vi "ACT_Loop.vi"() -> ()   [LabVIEW 2023, in "Thor-SwerveDrive_ACT.lvlib"]
uses:
  Thor-SwerveDrive_ACT.lvlib
  roboRIO Utilities/Global_STOP.vi
  ENUM_ACT_Action.ctl
  ENUM_ACT_State.ctl
  Global_CMD_ACT_Data In.vi
  Global_ACT_Data Out.vi
  Cluster_CMD_ACT_Data.ctl
  <vilib>/Rock Robotics/WPI/MotorControl/WPI_MotorControlType.ctl
  <vilib>/Rock Robotics/SystemInterfaces/DIO/FPGA_DIOPWMChannel.ctl
  <vilib>/Rock Robotics/WPI/PWM/WPI_PWMDeadband.ctl
  <vilib>/Rock Robotics/SystemInterfaces/DIO/FPGA_DIOChannel.ctl
  <vilib>/Rock Robotics/WPI/MotorControl/WPI_MotorControlDeviceRef.ctl
  Shared Code/TypeDefs/ENUM_Motor Index.ctl
  Shared Code/TypeDefs/ENUM_Swerve_CMD_Mode Select.ctl
  Type Defs/ENUM_Steer Mode Select.ctl
  Shared Code/TypeDefs/Cluster_CMD_Direction Data.ctl
  Shared Code/TypeDefs/Level_Velocity plus-minus 1.ctl
  Shared Code/TypeDefs/Dial_Compase heading unit circle CCW positive.ctl
  Shared Code/TypeDefs/Cluster_Module Velocity-Direction-Rotations.ctl
  Shared Code/TypeDefs/Cluster_Swerve 4 Steer and Velocity.ctl
  Shared Code/TypeDefs/Cluster_X-Y.ctl
  Type Defs/Cluster_Length and Width.ctl
  PigeonIMU/Global_SEN_Data Out.vi
  PigeonIMU/PigeonIMU_SEN.lvlib
  <vilib>/Rock Robotics/WPI/ThirdParty/Phoenix-LabVIEW/CANCoder/Controls/CTRE_Phoenix_CANcoder_DeviceRef.ctl
  <vilib>/Rock Robotics/WPI/ThirdParty/Phoenix-LabVIEW/Motor Controller/Controls/CTRE_Phoenix_MotorControl_ControlMode.ctl
  <vilib>/Rock Robotics/WPI/ThirdParty/Phoenix-LabVIEW/Motor Controller/Get/CTRE_Phoenix_MotorController_GetSelectedSensorData.vi
  Shared Code/TypeDefs/Cluster_Module Specific Config Data.ctl
  <vilib>/Rock Robotics/WPI/ThirdParty/Phoenix-LabVIEW/Motor Controller/Controls/CTRE_Phoenix_MotorControl_TalonFXInvertType.ctl
  <vilib>/Rock Robotics/WPI/ThirdParty/Phoenix-LabVIEW/Motor Controller/Controls/CTRE_Phoenix_MotorControl_NeutralMode.ctl
  Shared Code/TypeDefs/Cluster_Enable-Value DBL.ctl
  Shared Code/TypeDefs/Cluster_Swerve Module Drive Config Data.ctl
  Shared Code/TypeDefs/Cluster_PID Gains.ctl
  Shared Code/TypeDefs/Cluster_High-Low.ctl
  Shared Code/TypeDefs/Cluster_PID Config.ctl
  Shared Code/TypeDefs/Cluster_Swerve Module Azimuth Config Data.ctl
  Shared Code/TypeDefs/Cluster_Motion Magic Parameters.ctl
  Type Defs/NUM_Rotate Input.ctl
  Shared Code/TypeDefs/Cluster_Swerve Specific Data.ctl
  4adeeee4-476d-45d4-a5a4-571a9ae37a33.vi
  2c7c5537-7bdd-4d59-ad4f-3c8ee235c6a6.vi
  807b9100-2ea1-4d3f-8102-f0ab848f34e3.vi
  19b81104-80f8-498e-bad8-80b5a07e1603.vi
  e1bb1583-82cd-4173-857f-54dda67d13bd.vi
  9120009a-4733-4867-ae1d-0cf0254934b1.vi
  e3bd2e4a-1335-45b3-b961-e3cd167d7084.vi
  9ce11db1-6321-4cd7-bc1a-63dd18007c8f.vi
  Shared Code/TypeDefs/Cluster_FWD  REV Values.ctl
  Shared Code/TypeDefs/Cluster_Config Motor Output.ctl
  8c0680db-f6e2-43d9-8911-a02d1c4f353c.vi
  f7ff1910-59a6-4a5b-a4bc-add152f69b28.vi
  140e803e-7328-4941-96e6-52945a01db81.vi
  4178fa8d-7c82-4047-aba6-40e6de057a6a.vi
  2d114f5c-e136-49d5-a090-2a73a4719927.vi
  136452eb-6d18-483f-b532-0de35bf94788.vi
  Shared Code/TypeDefs/Cluster_Config_AutoRotate Data.ctl
  Shared Code/TypeDefs/Cluster_Config_AutoDrive Data.ctl
  Shared Code/TypeDefs/Cluster_Config_Balance Data.ctl
  eab307ff-2afe-4630-93b3-566b0cf5e78a.vi
  51c25ad4-39a0-4a24-89e8-b12740a342fe.vi
  Type Defs/Cluster_Pigeon Tilt Data.ctl
  Shared Code/TypeDefs/ENUM_Tilt State.ctl
  Shared Code/TypeDefs/Cluster_Config_SwerveParam Steer.ctl
  Shared Code/TypeDefs/Cluster_Config_SwerveParam Drive.ctl
  Shared Code/TypeDefs/Cluster_Config_Swerve Drive Parameters.ctl
  <vilib>/Rock Robotics/WPI/ThirdParty/Phoenix-LabVIEW/Motor Controller/Get/CTRE_Phoenix_MotorController_GetVoltage.vi
  <vilib>/Rock Robotics/WPI/ThirdParty/Phoenix-LabVIEW/CANCoder/Get/CTRE_Phoenix_CANcoder_GetSensorData.vi
  Shared Code/TypeDefs/Dial_Actual Direction.ctl
  Shared Code/TypeDefs/Cluster_Module Actual Settings.ctl
  Shared Code/TypeDefs/Cluster_Swerve Actual Settings.ctl
panel:
  out "x-y":dbl
  out "Velocity":dbl[](array[numeric])
  out "Velocity Out":dbl
  out "At Target":bool
  out "State":T1
  out "Balanced":bool
  in  "Balance Config":T2={"BalancePID Ver"=0, "PID"={"Gains"={"P"=4.0, "I"=0.0, "D"=50.0, "F"=0.0}, "Error Allowed"={"High"=0.01, "Low"=-0.01}, "I Zone"={"High"=10.0, "Low"=-10.0}, "Max Out"={"FWD"=0.44, "REV"=-0.44}, "Max I Accu"={"High"=100000.0, "Low"=-100000.0}, "CL Ramp Rate (S)"=0.01}} {"PID"."Max I Accu"."Low" format="%#.8f"; "PID"."Max I Accu"."High" format="%#.8f"; "PID"."Gains"."F" format="%#.8f"; "PID"."Gains"."D" format="%#.8f"; "PID"."Gains"."I" format="%#.8f"; "PID"."Gains"."P" format="%#.8f"; "PID"."Error Allowed"."Low" format="%#.8f"; "PID"."Error Allowed"."High" format="%#.8f"; "PID"."I Zone"."Low" format="%#.8f"; "PID"."I Zone"."High" format="%#.8f"; "PID"."Max Out"."REV" format="%.2f"; "PID"."Max Out"."FWD" format="%.2f"}
  out "At Angle":bool
  out "At Position":bool
  in  "Auto Rotate Config":T7={"AutoRotatePID Ver"=0, "PID Config"={"Gains"={"P"=0.005, "I"=0.001, "D"=0.0, "F"=0.0}, "Error Allowed"={"High"=0.05, "Low"=-0.05}, "I Zone"={"High"=0.25, "Low"=-0.25}, "Max Out"={"FWD"=1.0, "REV"=-1.0}, "Max I Accu"={"High"=100000.0, "Low"=-100000.0}, "CL Ramp Rate (S)"=0.002}} {"PID Config"."Max I Accu"."Low" format="%#.8f"; "PID Config"."Max I Accu"."High" format="%#.8f"; "PID Config"."Gains"."F" format="%#.8f"; "PID Config"."Gains"."D" format="%#.8f"; "PID Config"."Gains"."I" format="%#.8f"; "PID Config"."Gains"."P" format="%#.8f"; "PID Config"."Error Allowed"."Low" format="%#.8f"; "PID Config"."Error Allowed"."High" format="%#.8f"; "PID Config"."I Zone"."Low" format="%#.8f"; "PID Config"."I Zone"."High" format="%#.8f"; "PID Config"."Max Out"."REV" format="%.2f"; "PID Config"."Max Out"."FWD" format="%.2f"}
  out "PID Enabled":bool
  out "Auto Drive error":dbl
  in  "Auto PID Config":T8={"AutoDrivePID Ver"=0, "PID Config"={"Gains"={"P"=0.08, "I"=0.0, "D"=0.0, "F"=0.0}, "Error Allowed"={"High"=1.0, "Low"=-1.0}, "I Zone"={"High"=1.0, "Low"=-1.0}, "Max Out"={"FWD"=0.4, "REV"=-0.4}, "Max I Accu"={"High"=100000.0, "Low"=-100000.0}, "CL Ramp Rate (S)"=0.002}} {"PID Config"."Max I Accu"."Low" format="%#.8f"; "PID Config"."Max I Accu"."High" format="%#.8f"; "PID Config"."Gains"."F" format="%#.8f"; "PID Config"."Gains"."D" format="%#.8f"; "PID Config"."Gains"."I" format="%#.8f"; "PID Config"."Gains"."P" format="%#.8f"; "PID Config"."Error Allowed"."Low" format="%#.8f"; "PID Config"."Error Allowed"."High" format="%#.8f"; "PID Config"."I Zone"."Low" format="%#.8f"; "PID Config"."I Zone"."High" format="%#.8f"; "PID Config"."Max Out"."REV" format="%.2f"; "PID Config"."Max Out"."FWD" format="%.2f"}
  in  "Reset Distance":bool
  out "Calculated Position ft":dbl
  in  "Read Saved Config":bool
  out "Current Time":timestamp
  in  "Update Config":bool
  in  "Module Specific Data":T9={"SpecificData Ver"=0, "Data"=[{"Motor Pos"=enum."Left-Front", "CAN Bus"="", "Drive ID"=5, "Azimuth ID"=1, "CanCoder ID"=1, "CanCoder Offset"=14.502}, {"Motor Pos"=enum."Right-Front", "CAN Bus"="", "Drive ID"=6, "Azimuth ID"=2, "CanCoder ID"=2, "CanCoder Offset"=166.816}, {"Motor Pos"=enum."Right-Back", "CAN Bus"="", "Drive ID"=7, "Azimuth ID"=3, "CanCoder ID"=3, "CanCoder Offset"=50.273}, {"Motor Pos"=enum."Left-Back", "CAN Bus"="", "Drive ID"=8, "Azimuth ID"=4, "CanCoder ID"=4, "CanCoder Offset"=332.842}]}
  in  "Azimuth Config Data":T12={"ModuleAzimuth Ver"=0, "Output"={"Type"=enum."Counter-Clockwise", "Neutral"=enum."EEPROMSetting", "Max"={"FWD"=0.0, "REV"=1.0}, "Min"={"FWD"=0.0, "REV"=0.0}, "OL Ramp Rate (S)"=0.0, "Dead Band"=0.0}, "CL"={"Gains"={"P"=1.0, "I"=0.01, "D"=0.0, "F"=0.0}, "Error Allowed"={"High"=0.0, "Low"=0.0}, "I Zone"={"High"=10000.0, "Low"=-1000.0}, "Max Out"={"FWD"=1.0, "REV"=-1.0}, "Max I Accu"={"High"=10.0, "Low"=-10.0}, "CL Ramp Rate (S)"=0.0}, "MM"={"Cruise Velocity"=5000, "Acceleration"=5000}} {"Output"."Min"."REV" format="%.2f"; "Output"."Min"."FWD" format="%.2f"; "Output"."Max"."REV" format="%.2f"; "Output"."Max"."FWD" format="%.2f"; "CL"."Max I Accu"."Low" format="%#.8f"; "CL"."Max I Accu"."High" format="%#.8f"; "CL"."Gains"."F" format="%#.8f"; "CL"."Gains"."D" format="%#.8f"; "CL"."Gains"."I" format="%#.8f"; "CL"."Gains"."P" format="%#.8f"; "CL"."Error Allowed"."Low" format="%#.8f"; "CL"."Error Allowed"."High" format="%#.8f"; "CL"."I Zone"."Low" format="%#.8f"; "CL"."I Zone"."High" format="%#.8f"; "CL"."Max Out"."REV" format="%.2f"; "CL"."Max Out"."FWD" format="%.2f"}
  in  "Drive Config Data":T17={"ModuleDrive Ver"=0, "Output"={"Type"=enum."Counter-Clockwise", "Neutral"=enum."EEPROMSetting", "Max"={"FWD"=0.0, "REV"=0.0}, "Min"={"FWD"=0.0, "REV"=0.0}, "OL Ramp Rate (S)"=0.0, "Dead Band"=0.0}, "CL"={"Gains"={"P"=1.0, "I"=0.01, "D"=0.0, "F"=0.0}, "Error Allowed"={"High"=0.1, "Low"=-0.1}, "I Zone"={"High"=10.0, "Low"=-10.0}, "Max Out"={"FWD"=100.0, "REV"=-100.0}, "Max I Accu"={"High"=0.0, "Low"=0.0}, "CL Ramp Rate (S)"=0.0}, "VoltageComp"={"Enable"=FALSE, "Value"=0.0}} {"Output"."Min"."REV" format="%.2f"; "Output"."Min"."FWD" format="%.2f"; "Output"."Max"."REV" format="%.2f"; "Output"."Max"."FWD" format="%.2f"; "VoltageComp"."Value" format="%.1g"; "CL"."Max I Accu"."Low" format="%#.8f"; "CL"."Max I Accu"."High" format="%#.8f"; "CL"."Gains"."F" format="%#.8f"; "CL"."Gains"."D" format="%#.8f"; "CL"."Gains"."I" format="%#.8f"; "CL"."Gains"."P" format="%#.8f"; "CL"."Error Allowed"."Low" format="%#.8f"; "CL"."Error Allowed"."High" format="%#.8f"; "CL"."I Zone"."Low" format="%#.8f"; "CL"."I Zone"."High" format="%#.8f"; "CL"."Max Out"."REV" format="%.2f"; "CL"."Max Out"."FWD" format="%.2f"}
  out "Drive Control Mode":T19 items=["PercentOutput"=0, "Position"=1, "Velocity"=2, "Current"=3, "Follower"=5, "MotionProfile"=6, "MotionMagic"=7, "MotionProfileArc"=10, "Disabled"=15]
  out "MOTOR-POSITION":dbl[](array[numeric])
  out "CAN-POSITION":dbl[](array[numeric])
  out "RAW":dbl[](array[numeric])
  out "Yaw":T20 scale format="%.3f"
  out "Swerve SET Actual":T21 {"Back Right"."Direction" scale format="%.3f"; "Back Right"."Velocity" format="%.2f"; "Back Left"."Direction" scale format="%.3f"; "Back Left"."Velocity" format="%.2f"; "Front Left"."Direction" scale format="%.3f"; "Front Left"."Velocity" format="%.2f"; "Front Right"."Direction" scale format="%.3f"; "Front Right"."Velocity" format="%.2f"}
  out "calc time":dbl
  out "Swerve Set":T24 {"Back Right"."Angle" scale format="%.3f"; "Back Right"."Velocity" scale=-1.0..1.0 scale format="%.1f"; "Back Left"."Angle" scale format="%.3f"; "Back Left"."Velocity" scale=-1.0..1.0 scale format="%.1f"; "Front Left"."Angle" scale format="%.3f"; "Front Left"."Velocity" scale=-1.0..1.0 scale format="%.1f"; "Front Right"."Angle" scale format="%.3f"; "Front Right"."Velocity" scale=-1.0..1.0 scale format="%.1f"}
  out "Max Velocity(CP100ms)":dbl=200.0
  out "Steer Mode":T27
  out "Max Tranlation FPS":dbl=2.0
  out "Calculated Position Values":i32[](array[numeric])
  in  "Stream":bool
  out "Input CMD":T28 {"Auto Angle" scale format="%.3f"; "Direction"."Rotate(Yaw) CCW 1 CW -1" scale=1.0..-1.0; "Direction"."Traverse"."Angle" scale format="%.3f"; "Direction"."Traverse"."Velocity" scale=-1.0..1.0 scale format="%.1f"}
  out "Cycle Time (S)":dbl format="%.3g"
  # "Tune Output\nto 1023 Max"
  # "Tune to Output\nto 1023 Max"
  # "\"Front\" of Robot"
  # "X"
  # "+CCW"
  # "Y"
  # "(0,0)"
  # "\"Front\" of Robot"
  # "Right Hand Rule"
  # "X"
  # "+CCW"
  # "Y"
  # "(0,0)"
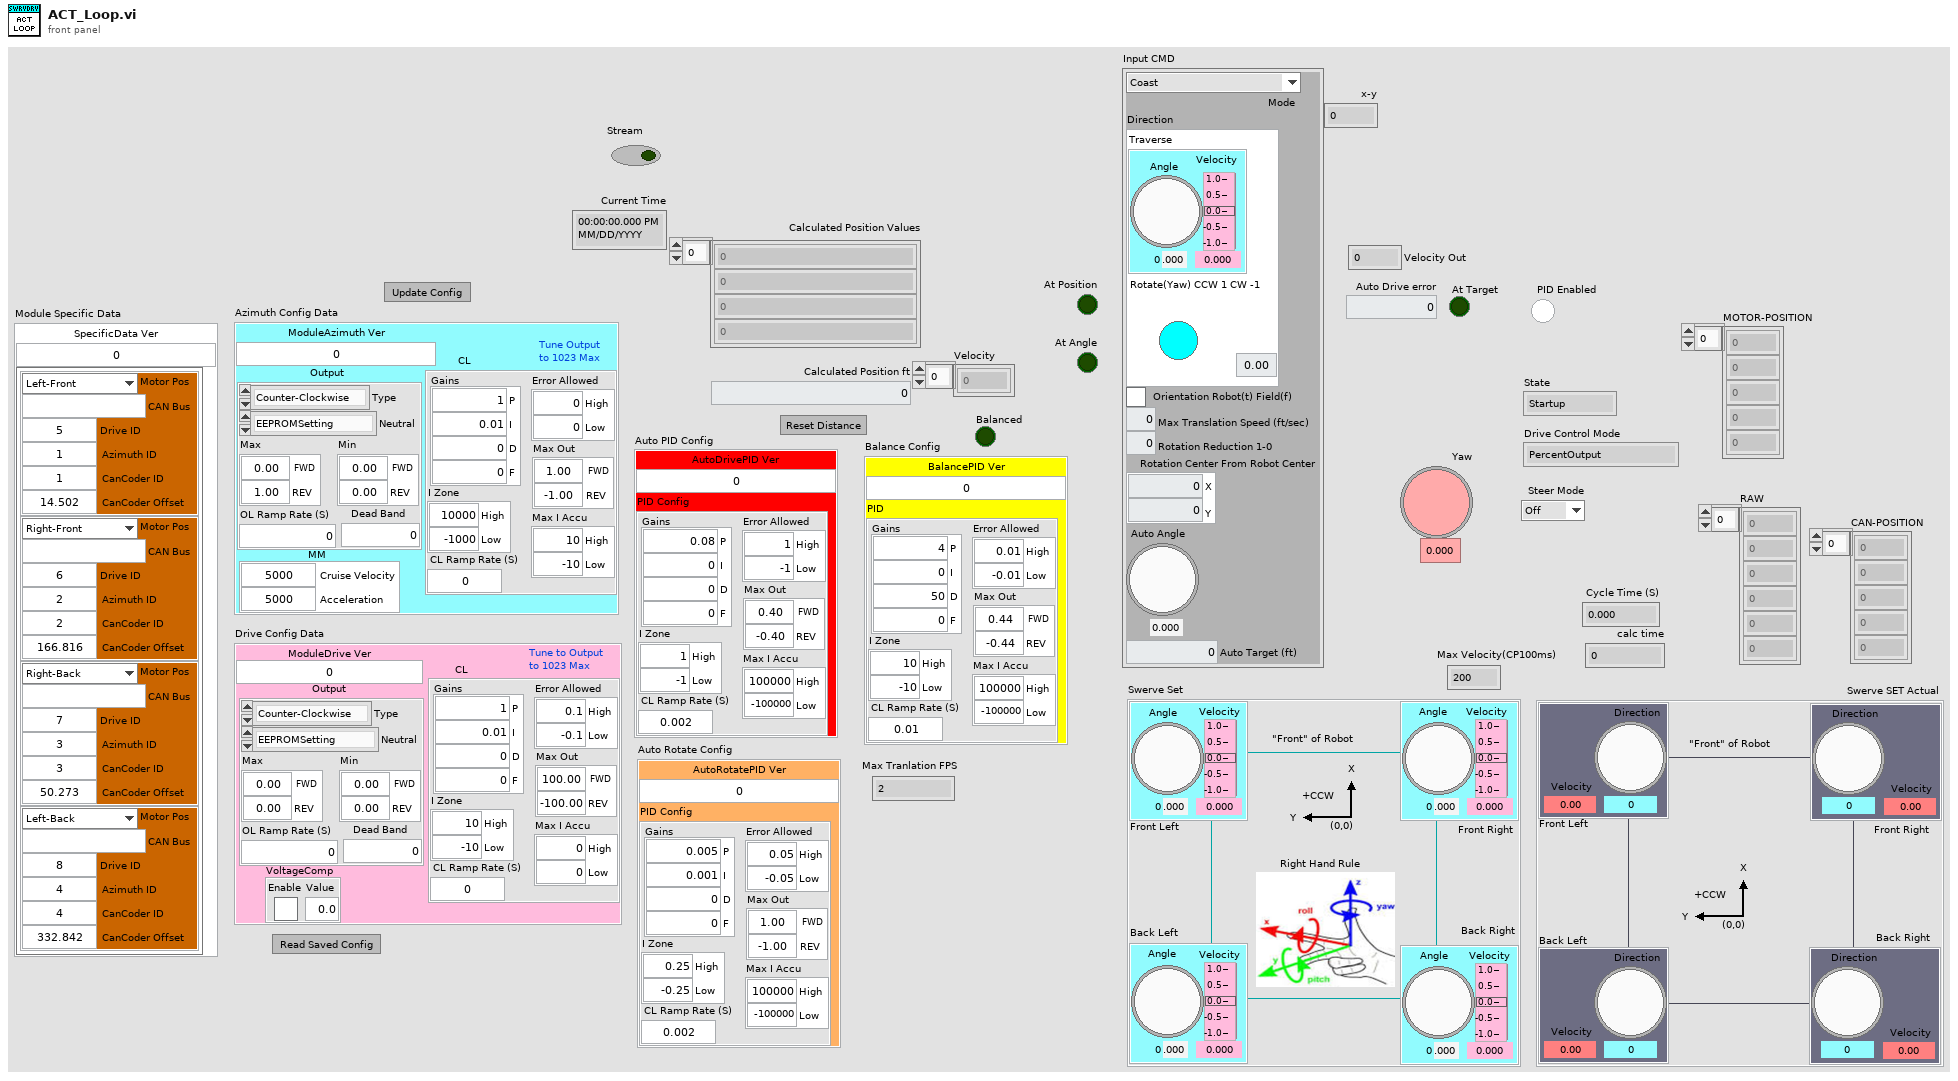
[diagram p1: front panel]
types:
  T1 = typedef "Thor-SwerveDrive_ACT.lvlib/ENUM_ACT_State.ctl" = enum16{"Startup", "Configuring", "Moving", "Coasting", "Shutdown", "Autoing", "Balancing", "Braking", "Locking Wheels"}
  T2 = typedef "Cluster_Config_Balance Data.ctl" = cluster{"BalancePID Ver":u64, "PID":T3}
  T3 = typedef "Cluster_PID Config.ctl" = cluster{"Gains":T4, "Error Allowed":T5, "I Zone":T5, "Max Out":T6, "Max I Accu":T5, "CL Ramp Rate (S)":dbl}
  T4 = typedef "Cluster_PID Gains.ctl" = cluster{"P":dbl, "I":dbl, "D":dbl, "F":dbl}
  T5 = typedef "Cluster_High-Low.ctl" = cluster{"High":dbl, "Low":dbl}
  T6 = typedef "Cluster_FWD  REV Values.ctl" = cluster{"FWD":dbl, "REV":dbl}
  T7 = typedef "Cluster_Config_AutoRotate Data.ctl" = cluster{"AutoRotatePID Ver":u64, "PID Config":T3}
  T8 = typedef "Cluster_Config_AutoDrive Data.ctl" = cluster{"AutoDrivePID Ver":u64, "PID Config":T3}
  T9 = typedef "Cluster_Swerve Specific Data.ctl" = cluster{"SpecificData Ver":u64, "Data":T10[]}
  T10 = typedef "Cluster_Module Specific Config Data.ctl" = cluster{"Motor Pos":T11, "CAN Bus":string, "Drive ID":u8, "Azimuth ID":u8, "CanCoder ID":u8, "CanCoder Offset":dbl}
  T11 = typedef "ENUM_Motor Index.ctl" = enum16{"Left-Front", "Right-Front", "Left-Back", "Right-Back"}
  T12 = typedef "Cluster_Swerve Module Azimuth Config Data.ctl" = cluster{"ModuleAzimuth Ver":u64, "Output":T13, "CL":T3, "MM":T16}
  T13 = typedef "Cluster_Config Motor Output.ctl" = cluster{"Type":T14, "Neutral":T15, "Max":T6, "Min":T6, "OL Ramp Rate (S)":dbl, "Dead Band":dbl}
  T14 = typedef "CTRE_Phoenix_MotorControl_TalonFXInvertType.ctl" = enum16{"Counter-Clockwise", "Clockwise"}
  T15 = typedef "CTRE_Phoenix_MotorControl_NeutralMode.ctl" = enum8{"EEPROMSetting", "Override to Coast", "Override to Brake"}
  T16 = typedef "Cluster_Motion Magic Parameters.ctl" = cluster{"Cruise Velocity":i32, "Acceleration":i32}
  T17 = typedef "Cluster_Swerve Module Drive Config Data.ctl" = cluster{"ModuleDrive Ver":u64, "Output":T13, "CL":T3, "VoltageComp":T18}
  T18 = typedef "Cluster_Enable-Value DBL.ctl" = cluster{"Enable":bool, "Value":dbl}
  T19 = typedef "CTRE_Phoenix_MotorControl_ControlMode.ctl" = u16
  T20 = typedef "Dial_Compase heading unit circle CCW positive.ctl" = dbl
  T21 = typedef "Cluster_Swerve Actual Settings.ctl" = cluster{"Front Right":T22, "Front Left":T22, "Back Left":T22, "Back Right":T22}
  T22 = typedef "Cluster_Module Actual Settings.ctl" = cluster{"Velocity":dbl, "Direction":T23, "Encoder":dbl}
  T23 = typedef "Dial_Actual Direction.ctl" = dbl
  T24 = typedef "Cluster_Swerve 4 Steer and Velocity.ctl" = cluster{"Front Right":T25, "Front Left":T25, "Back Left":T25, "Back Right":T25}
  T25 = typedef "Cluster_Module Velocity-Direction-Rotations.ctl" = cluster{"Velocity":T26, "Angle":T20, "Rotations Count":dbl}
  T26 = typedef "Level_Velocity plus-minus 1.ctl" = dbl
  T27 = typedef "ENUM_Steer Mode Select.ctl" = enum16{"Off", "Hold", "Steer"}
  T28 = typedef "Thor-SwerveDrive_ACT.lvlib/Cluster_CMD_ACT_Data.ctl" = cluster{"Mode":T29, "Direction":T30, "Orientation Robot(t) Field(f)":bool, "Max Translation Speed (ft/sec)":dbl, "Rotation Reduction 1-0":dbl, "Rotation Center From Robot Center":T32, "Auto Angle":T20, "Auto Target (ft)":dbl}
  T29 = typedef "ENUM_Swerve_CMD_Mode Select.ctl" = enum16{"Coast", "Manual", "Auto Trans Auto Rotate", "Manual Trans Auto Rotate", "Balance", "Stop Brake", "Lock Wheels"}
  T30 = typedef "Cluster_CMD_Direction Data.ctl" = cluster{"Traverse":T25, "Rotate(Yaw) CCW 1 CW -1":T31}
  T31 = typedef "NUM_Rotate Input.ctl" = dbl
  T32 = typedef "Cluster_X-Y.ctl" = cluster{"X":dbl, "Y":dbl}
  T33 = typedef "Cluster_Length and Width.ctl" = cluster{"Length":dbl, "Width":dbl}
  T34 = typedef "Cluster_Config_Swerve Drive Parameters.ctl" = cluster{"SwerveParam Ver":u64, "Frame":T33, "Steer":T35, "Drive":T36}
  T35 = typedef "Cluster_Config_SwerveParam Steer.ctl" = cluster{"CPR":dbl}
  T36 = typedef "Cluster_Config_SwerveParam Drive.ctl" = cluster{"CPR":dbl, "RevMotor/Wheel":dbl, "Wheel Diameter (in)":dbl}
  T37 = typedef "Cluster_Pigeon Tilt Data.ctl" = cluster{"Angle":dbl, "Tilt Changing":bool, "BACK UP":bool, "Tilt":dbl, "Disable":bool, "BACK DOWN":bool, "Tilt State":T38}
  T38 = typedef "ENUM_Tilt State.ctl" = enum16{"Unknown", "Level", "Angle UP from Level", "Level from Angle Up", "Angle Down from Level", "Level from Angle Down"}
  T39 = typedef "CTRE_Phoenix_CANcoder_DeviceRef.ctl" = cluster{"DeviceStatus":errorcluster, "Device Number":u8, "Handle":u64, "UsageFrame":u32, "Library Path":path}
  T40 = typedef "WPI_MotorControlDeviceRef.ctl" = cluster{"DeviceStatus":errorcluster, "Type":T41, "PWM":cluster{"PWM Channel":T42, "DeadBand":T43}, "CAN":cluster{"Device Number":u8, "SetOutput VI Ref":variant, "GetOutput VI Ref":variant, "Enable VI Ref":variant, "Disable VI Ref":variant, "Data":variant}, "Invert":bool, "DIO PWM":cluster{"PWM \"Enable\" Channel":T42, "DIOChannel":T44, "PWM Rate":dbl}}
  T41 = typedef "WPI_MotorControlType.ctl" = enum16{"PWM", "CAN", "DIO PWM"}
  T42 = typedef "FPGA_DIOPWMChannel.ctl" = enum8{"PWM 0", "PWM 1", "PWM 2", "PWM 3", "PWM 4", "PWM 5", "PWM 6", "PWM 7", "PWM 8", "PWM 9", "PWM MXP 0", "PWM MXP 1", "PWM MXP 2", "PWM MXP 3", "PWM MXP 4", "PWM MXP 5", "PWM MXP 6", "PWM MXP 7", "PWM MXP 8", "PWM MXP 9", "Invalid"}
  T43 = typedef "WPI_PWMDeadband.ctl" = cluster{"Name":string, "maxPositivePwm":i32, "minPositivePwm":i32, "centerPwm":i32, "maxNegativePwm":i32, "minNegativePwm":i32, "angularRange":u16}
  T44 = typedef "FPGA_DIOChannel.ctl" = enum8{"DIO 0", "DIO 1", "DIO 2", "DIO 3", "DIO 4", "DIO 5", "DIO 6", "DIO 7", "DIO 8", "DIO 9", "DIO MXP 0", "DIO MXP 1", "DIO MXP 2", "DIO MXP 3", "DIO MXP 4", "DIO MXP 5", "DIO MXP 6", "DIO MXP 7", "DIO MXP 8", "DIO MXP 9", "DIO MXP 10", "DIO MXP 11", "DIO MXP 12", "DIO MXP 13", "DIO MXP 14", "DIO MXP 15", "SPI Port CS1", "SPI Port CS2", "SPI Port CS3", "SPI Port MISO", "SPI Port MOSI", "Invalid"}
  T45 = cluster{"Motor List":T11[], "Drive Refs":T40[], "Steer Refs":T40[], "State":T1, "Previous State":T1, "Current Time":timestamp, "Previous Time":timestamp, "Start Time":timestamp, "Target Time (ms)":u32, "Cycle Time(S)":dbl, "ACT Input":T28, "Drive PID Slot":i32, "Steer Position Values":dbl[], "Drive Velocity Values":dbl[], "Steer Position Times":dbl[], "Drive Velocity Times":dbl[], "Stream":bool, "Drive Output Times":dbl[], "Drive Output Values":dbl[], "Steer Mode":T27, "Max Velocity CP100ms":dbl, "Swerve Set":T24, "calc Start Time":dbl, "Compass Heading":T20, "CANCoder Refs":T39[], "Drive Control Mode":T19, "Specific Config":T9, "Azimuth Config":T12, "Drive Config":T17, "Team Folder":path, "Update Display":bool, "Rotation PID Config":T7, "Drive Position Offsets":i32[], "Drive Position Values":i32[], "Calculated Position (ft)":dbl, "Auto PID Config":T8, "At Position":bool, "At Angle":bool, "Balance Config ":T2, "Reset Balance":bool, "Tilt Data":T37, "Balanced":bool, "New Cmd":bool, "SwerveConfig ":T34}
  T46 = typedef "Thor-SwerveDrive_ACT.lvlib/ENUM_ACT_Action.ctl" = enum16{"Set Move from Values", "Swerve Config Drive Read ", "Swerve Config Azimuth Read", "No Action", "Reset Time", "Set to Coast", "Record Data", "Swerve Open Only", "Swerve Config ALL Update", "Swerve Config Azimuth Update", "Swerve Config Drive Update", "Swerve Config From FP Update", "File Config ALL Save", "File Config ALL Read", "Save Position Offsets", "Drive Auto PID", "Balance", "Brake", "Lock"}
  T47 = typedef "SwerveDrive_ACT.lvlib/Cluster_CMD_ACT_Data.ctl" = cluster{"Mode":T29, "Direction":T30, "Orientation Robot(t) Field(f)":bool, "Max Translation Speed (ft/sec)":dbl, "Rotation Reduction 1-0":dbl, "Rotation Center From Robot Center":T32, "Auto Angle":T20, "Auto Target (ft)":dbl}
  T48 = typedef "Cluster_Unity Yaw-Pitch-Roll.ctl" = cluster{"Yaw":T20, "Pitch":T20, "Roll":T20}
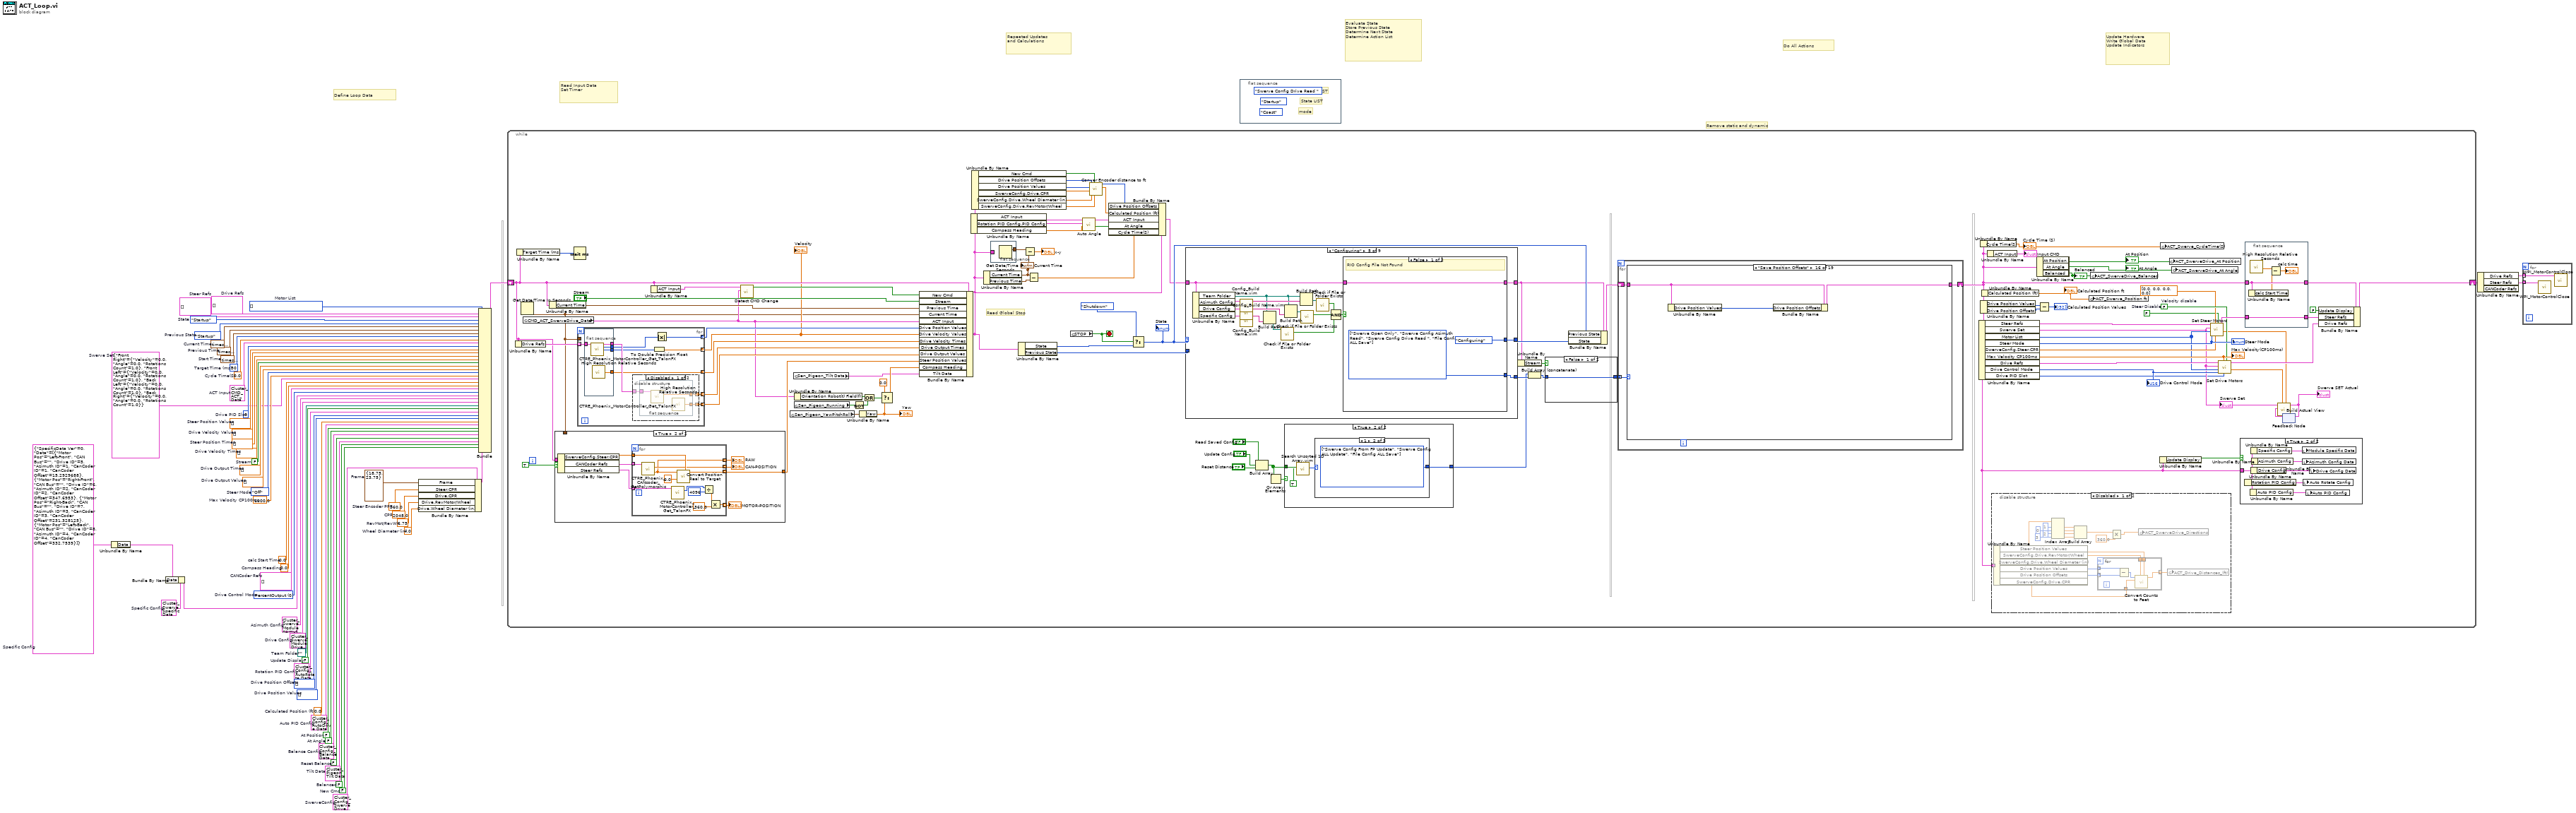
[diagram p0: block diagram]
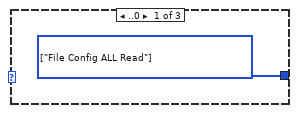
[diagram p4: hidden frame]
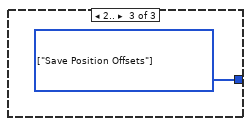
[diagram p5: hidden frame]
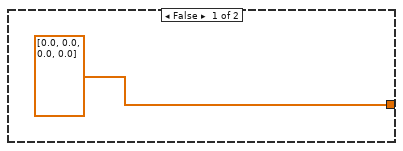
[diagram p7: hidden frame]
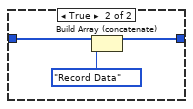
[diagram p9: hidden frame]
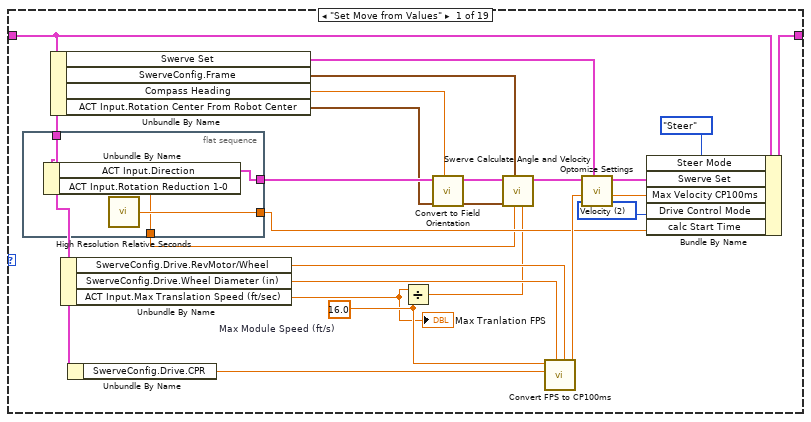
[diagram p10: hidden frame]
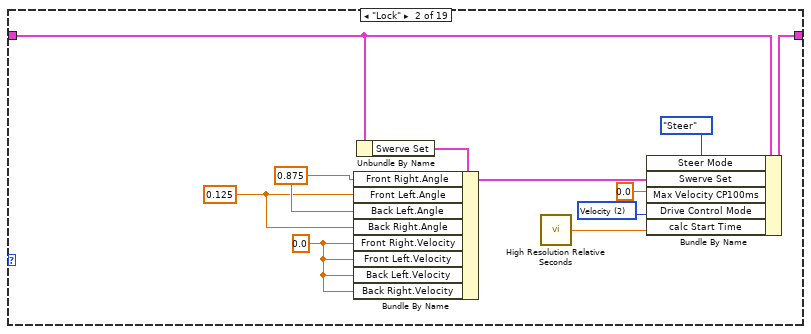
[diagram p11: hidden frame]
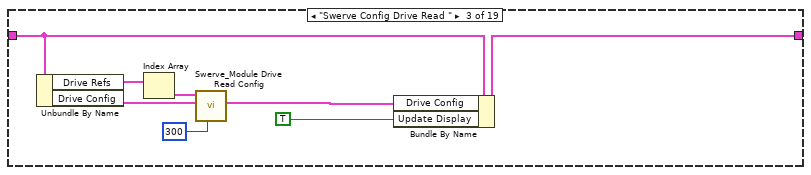
[diagram p12: hidden frame]
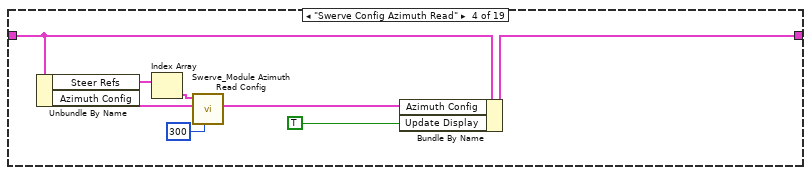
[diagram p13: hidden frame]
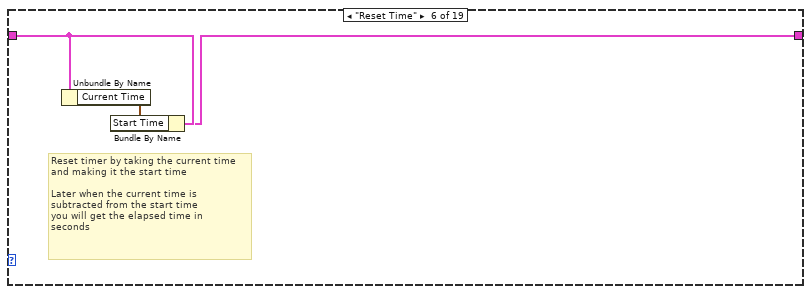
[diagram p15: hidden frame]
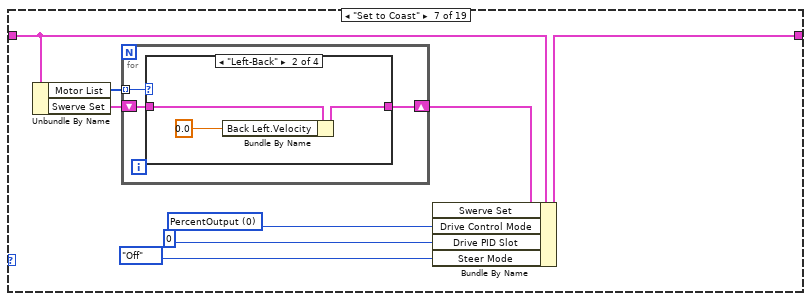
[diagram p16: hidden frame]
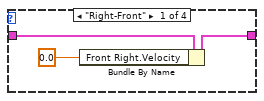
[diagram p17: hidden frame]
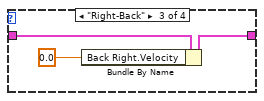
[diagram p18: hidden frame]
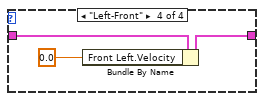
[diagram p19: hidden frame]
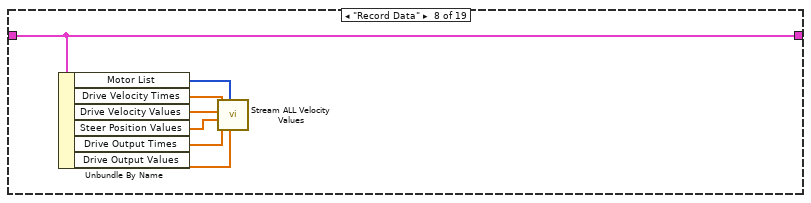
[diagram p20: hidden frame]
diagram:
  w1 = 4.0  # Wheel Diameter (in)
  w2 = 6.75  # RevMot/RevWh
  w3 = 2048.0  # CPR
  w4 = 360.0  # Steer Encoder PPR
  w5 = T33 {"Length"=18.75, "Width"=23.75}  # Frame
  w7 = T34 {"SwerveParam Ver"=0, "Frame"={"Length"=18.75, "Width"=23.75}, "Steer"={"CPR"=360.0}, "Drive"={"CPR"=2048.0, "RevMotor/Wheel"=6.75, "Wheel Diameter (in)"=4.0}}  # SwerveConfig
  w8 = FALSE  # New Cmd
  w9 = FALSE  # Balanced
  w10 = T37 {"Angle"=-0.0030517578125, "Tilt Changing"=FALSE, "BACK UP"=FALSE, "Tilt"=0.0, "Disable"=FALSE, "BACK DOWN"=FALSE, "Tilt State"=enum."Unknown"}  # Tilt Data
  w11 = FALSE  # Reset Balance
  w12 = T2 {"BalancePID Ver"=0, "PID"={"Gains"={"P"=4.0, "I"=0.0, "D"=50.0, "F"=0.0}, "Error Allowed"={"High"=0.01, "Low"=-0.01}, "I Zone"={"High"=10.0, "Low"=-10.0}, "Max Out"={"FWD"=0.44, "REV"=-0.44}, "Max I Accu"={"High"=100000.0, "Low"=-100000.0}, "CL Ramp Rate (S)"=0.01}}  # Balance Config
  w13 = FALSE  # At Angle
  w14 = FALSE  # At Position
  w15 = T8 {"AutoDrivePID Ver"=0, "PID Config"={"Gains"={"P"=0.0065, "I"=0.001, "D"=0.0, "F"=0.0}, "Error Allowed"={"High"=0.1, "Low"=-0.1}, "I Zone"={"High"=2.0, "Low"=-2.0}, "Max Out"={"FWD"=1.0, "REV"=-1.0}, "Max I Accu"={"High"=100000.0, "Low"=-100000.0}, "CL Ramp Rate (S)"=0.002}}  # Auto PID Config
  w16 = 0.0  # Calculated Position (ft)
  w17 = i32[] []  # Drive Position Values
  w18 = i32[] []  # Drive Position Offsets
  w19 = T7 {"AutoRotatePID Ver"=0, "PID Config"={"Gains"={"P"=0.08, "I"=0.0, "D"=0.0, "F"=0.0}, "Error Allowed"={"High"=1.0, "Low"=1.0}, "I Zone"={"High"=1.0, "Low"=1.0}, "Max Out"={"FWD"=0.4, "REV"=-0.4}, "Max I Accu"={"High"=100000.0, "Low"=-100000.0}, "CL Ramp Rate (S)"=0.0}}  # Rotation PID Config
  w21 = T9 {"SpecificData Ver"=0, "Data"=[{"Motor Pos"=enum."Left-Front", "CAN Bus"="", "Drive ID"=5, "Azimuth ID"=1, "CanCoder ID"=1, "CanCoder Offset"=15.2929688}, {"Motor Pos"=enum."Right-Front", "CAN Bus"="", "Drive ID"=6, "Azimuth ID"=2, "CanCoder ID"=2, "CanCoder Offset"=347.6953}, {"Motor Pos"=enum."Right-Back", "CAN Bus"="", "Drive ID"=7, "Azimuth ID"=3, "CanCoder ID"=3, "CanCoder Offset"=231.328125}, {"Motor Pos"=enum."Left-Back", "CAN Bus"="", "Drive ID"=8, "Azimuth ID"=4, "CanCoder ID"=4, "CanCoder Offset"=332.7539}]}  # Specific Config
  w25 = FALSE  # Update Display
  w23 = T9 {"SpecificData Ver"=0, "Data"=[{"Motor Pos"=enum."Left-Front", "CAN Bus"="", "Drive ID"=5, "Azimuth ID"=1, "CanCoder ID"=1, "CanCoder Offset"=14.502}, {"Motor Pos"=enum."Right-Front", "CAN Bus"="", "Drive ID"=6, "Azimuth ID"=2, "CanCoder ID"=2, "CanCoder Offset"=166.816}, {"Motor Pos"=enum."Right-Back", "CAN Bus"="", "Drive ID"=7, "Azimuth ID"=3, "CanCoder ID"=3, "CanCoder Offset"=50.273}, {"Motor Pos"=enum."Left-Back", "CAN Bus"="", "Drive ID"=8, "Azimuth ID"=4, "CanCoder ID"=4, "CanCoder Offset"=332.842}]}  # Specific Config
  w26 = path ""  # Team Folder
  w27 = T17 {"ModuleDrive Ver"=0, "Output"={"Type"=enum."Counter-Clockwise", "Neutral"=enum."EEPROMSetting", "Max"={"FWD"=0.0, "REV"=0.0}, "Min"={"FWD"=0.0, "REV"=0.0}, "OL Ramp Rate (S)"=0.0, "Dead Band"=0.0}, "CL"={"Gains"={"P"=1.0, "I"=0.01, "D"=0.0, "F"=0.0}, "Error Allowed"={"High"=0.1, "Low"=-0.1}, "I Zone"={"High"=10.0, "Low"=-10.0}, "Max Out"={"FWD"=100.0, "REV"=-100.0}, "Max I Accu"={"High"=0.0, "Low"=0.0}, "CL Ramp Rate (S)"=0.0}, "VoltageComp"={"Enable"=FALSE, "Value"=0.0}}  # Drive Config
  w28 = T12 {"ModuleAzimuth Ver"=0, "Output"={"Type"=enum."Clockwise", "Neutral"=enum."Override to Brake", "Max"={"FWD"=1.0, "REV"=2.0}, "Min"={"FWD"=0.0, "REV"=0.0}, "OL Ramp Rate (S)"=0.0, "Dead Band"=0.0}, "CL"={"Gains"={"P"=1.0, "I"=-1.0, "D"=0.0, "F"=0.0}, "Error Allowed"={"High"=0.0, "Low"=0.0}, "I Zone"={"High"=0.0, "Low"=0.0}, "Max Out"={"FWD"=0.0, "REV"=0.0}, "Max I Accu"={"High"=1.0, "Low"=-1.0}, "CL Ramp Rate (S)"=0.0}, "MM"={"Cruise Velocity"=0, "Acceleration"=0}}  # Azimuth Config
  w29 = T11[] [] items=["Left-Front", "Right-Front", "Left-Back", "Right-Back"]  # Motor List
  w30 = T19 0 items=["PercentOutput"=0, "Position"=1, "Velocity"=2, "Current"=3, "Follower"=5, "MotionProfile"=6, "MotionMagic"=7, "MotionProfileArc"=10, "Disabled"=15]  # Drive Control Mode
  w31 = T39[] []  # CANCoder Refs
  w32 = T20 0.0  # Compass Heading
  w33 = 0.0  # calc Start Time
  w34 = T24 {"Front Right"={"Velocity"=0.0, "Angle"=0.0, "Rotations Count"=1.0}, "Front Left"={"Velocity"=0.0, "Angle"=0.0, "Rotations Count"=1.0}, "Back Left"={"Velocity"=0.0, "Angle"=0.0, "Rotations Count"=1.0}, "Back Right"={"Velocity"=0.0, "Angle"=0.0, "Rotations Count"=1.0}}  # Swerve Set
  w35 = 6000.0  # Max Velocity CP100ms
  w36 = ENUM_Steer_Mode_Select."Off"  # Steer Mode
  w37 = dbl[] []  # Drive Output Values
  w38 = dbl[] []  # Drive Output Times
  w39 = FALSE  # Stream
  w40 = dbl[] []  # Drive Velocity Times
  w41 = dbl[] []  # Steer Position Times
  w42 = dbl[] []  # Drive Velocity Values
  w43 = dbl[] []  # Steer Position Values
  w46 = 0  # Drive PID Slot
  w47 = T40[] []  # Drive Refs
  w48 = T40[] []  # Steer Refs
  w50 = 0.0  # Cycle Time(S)
  w51 = ENUM_ACT_State."Startup"  # Previous State
  w52 = timestamp(0 s since 1904-01-01)  # Previous Time
  w53 = u32 50  # Target Time (ms)
  w54 = T28 {"Mode"=enum."Coast", "Direction"={"Traverse"={"Velocity"=0.0, "Angle"=0.0, "Rotations Count"=0.0}, "Rotate(Yaw) CCW 1 CW -1"=0.0}, "Orientation Robot(t) Field(f)"=FALSE, "Max Translation Speed (ft/sec)"=0.0, "Rotation Reduction 1-0"=0.0, "Rotation Center From Robot Center"={"X"=0.0, "Y"=0.0}, "Auto Angle"=0.0, "Auto Target (ft)"=0.0}  # ACT Input
  w55 = timestamp(0 s since 1904-01-01)  # Start Time
  w56 = timestamp(0 s since 1904-01-01)  # Current Time
  w57 = ENUM_ACT_State."Startup"  # State
  # "Remove static and dynamic"
  # "Define Loop Data"
  # "Repeated Updates\nand Calculations"
  # "Read Input Data\nSet Timer"
  # "Evaluate State\nStore Previous State\nDetermine Next State\nDetermine Action List"
  # "Do All Actions"
  # "Update Hardware\nWrite Global Data\nUpdate Indicators"
  n1 = Unbundle By Name(w21) -> ("Data"=w20:T10[])
  n2 = Bundle By Name(cluster=w23, "Data"=w20) -> (w22:T9)
  n3 = Bundle By Name(cluster=w7, "Frame"=w5, "Steer.CPR"=w4, "Drive.CPR"=w3, "Drive.RevMotor/Wheel"=w2, "Drive.Wheel Diameter (in)"=w1) -> (w6:T34)
  n4 = Bundle("Motor List"=w29, "Drive Refs"=w47, "Steer Refs"=w48, "State"=w57, "Previous State"=w51, "Current Time"=w56, "Previous Time"=w52, "Start Time"=w55, "Target Time (ms)"=w53, "Cycle Time(S)"=w50, "ACT Input"=w54, "Drive PID Slot"=w46, "Steer Position Values"=w43, "Drive Velocity Values"=w42, "Steer Position Times"=w41, "Drive Velocity Times"=w40, "Stream"=w39, "Drive Output Times"=w38, "Drive Output Values"=w37, "Steer Mode"=w36, "Max Velocity CP100ms"=w35, "Swerve Set"=w34, "calc Start Time"=w33, "Compass Heading"=w32, "CANCoder Refs"=w31, "Drive Control Mode"=w30, "Specific Config"=w22, "Azimuth Config"=w28, "Drive Config"=w27, "Team Folder"=w26, "Update Display"=w25, "Rotation PID Config"=w19, "Drive Position Offsets"=w18, "Drive Position Values"=w17, "Calculated Position (ft)"=w16, "Auto PID Config"=w15, "At Position"=w14, "At Angle"=w13, "Balance Config"=w12, "Reset Balance"=w11, "Tilt Data"=w10, "Balanced"=w9, "New Cmd"=w8, "SwerveConfig"=w6) -> (w24:T45)  [unwired: 1 in]
  n5 = while {
    shift-right: [w142] -> w49
    shift-left: w24 -> [w71]
    stop <- w151 stop-if-true
    w76 = FALSE  # Steer Disable
    w119 = FALSE  # Velocity disable
    # "Read Global Stop"
    n6 = Unbundle By Name(w71) -> ("Drive Refs"=w129:T40[])
    n7 = Unbundle By Name(w71) -> ("Target Time (ms)"=w148:u32)
    n8 = Get Date/Time In Seconds() -> (seconds since 1Jan1904=w58:timestamp)
    n9 = global read "Global_CMD_ACT_Data In.vi" "CMD_ACT_SwerveDrive_Data"() -> (w72:T47)
    n10 = Unbundle By Name(w71) -> ("Current Time"=w147:timestamp)
    n11 = case shown="True" TRUE {
      tunnel: [dbl[] [0.0, 0.0, 0.0, 0.0] w207] -> w130
      tunnel: w71 -> [_ w206]
      tunnel: w58 -> [_ _]
      frame False {
      }
      frame True {
        n12 = Unbundle By Name(w206) -> ("SwerveConfig.Steer.CPR"=w204:dbl, "CANCoder Refs"=w205:T39[], "Steer Refs"=w201:T40[])
        n13 = for {
          tunnel: w205 -> [w217] mode=indexing
          tunnel: [w219] -> w207 mode=indexing
          tunnel: w204 -> [w218]
          tunnel: [w208] -> w203 mode=indexing
          tunnel: [w215] -> w202 mode=indexing
          tunnel: w201 -> [w214] mode=indexing
          tunnel: [w209] -> w200 mode=indexing
          n14 = call-poly <vilib>:"CTRE_Phoenix_CANcoder_GetPolymorphic.vi"("CTRE_CANcoder_DeviceRef"=w217) -> ("Position"=w215:dbl, "Absolute Position"=w208:dbl)  [unwired: 10 in, 3 out]
          n15 = call-poly <vilib>:"CTRE_Phoenix_MotorController_Get_TalonFX.vi"("PhoenixMotorControlDevRef"=w214) -> ("Position (Raw Sensor Units)"=w213:i32)  [unwired: 11 in, 3 out]
          n16 = call "Convert Position Real to Target.vi"("PPR"=w218, "Zero Value"=0.0, "Real Position"=w208) -> ("Position (0-1)"=w219:dbl)  [unwired: 8 in]
          n17 = Divide(x=w213, y=4096) -> (x/y=w211:dbl)
          n18 = Multiply(x=w211, y=360.0) -> (x*y=w209:dbl)
        }
        "RAW" <- w203
        "CAN-POSITION" <- w202
        "MOTOR-POSITION" <- w200
      }
    }
    n19 = Wait (ms)(milliseconds to wait=w148) -> ()  [unwired: 1 out]
    n20 = for {
      tunnel: w129 -> [w228] mode=indexing
      tunnel: [w222] -> w63 mode=indexing
      tunnel: [w224] -> w137 mode=indexing
      tunnel: [w226] -> w135 mode=indexing
      tunnel: [w225] -> w134 mode=indexing
      tunnel: [w220] -> w96 mode=indexing
      tunnel: w58 -> [_]
      n21 = flat-sequence {
        tunnel: w228 -> [w239]
        tunnel: [w238] -> w223
        tunnel: [w237] -> w227
        tunnel: [w236] -> w224
        tunnel: [w235] -> w221
        frame #0 {
          n22 = call-poly <vilib>:"CTRE_Phoenix_MotorController_Get_TalonFX.vi"("PhoenixMotorControlDevRef"=w239) -> ("PhoenixMotorControlDevRef"=w237:T40, "Position (Raw Sensor Units)"=w235:i32, "Velocity (Raw Sensor Units per 100 ms)"=w238:i32)  [unwired: 11 in, 1 out]
          n23 = call <vilib>:"High Resolution Relative Seconds.vi"() -> ("relative seconds"=w236:dbl)
        }
      }
      n24 = disable-structure shown="Disabled" {
        disable-tunnel: w227 -> [w231 _]
        disable-tunnel: [w230 _] -> w226
        disable-tunnel: [w229 _] -> w225
        frame Disabled {
          n25 = flat-sequence {
            tunnel: w231 -> [w234]
            tunnel: [w233] -> w230
            tunnel: [w232] -> w229
            frame #0 {
              n26 = call-poly <vilib>:"CTRE_Phoenix_MotorController_Get_TalonFX.vi"("PhoenixMotorControlDevRef"=w234) -> ("Percent Output"=w233:dbl)  [unwired: 10 in, 4 out]
              n27 = call <vilib>:"High Resolution Relative Seconds.vi"() -> ("relative seconds"=w232:dbl)
            }
          }
        }
        frame Enabled {
        }
      }
      n28 = To Double Precision Float(number=w223) -> (double precision float=w222:dbl)
      n29 = Absolute Value(x=w221) -> (abs(x)=w220:i32)
    }
    "Velocity" <- w63
    n30 = Unbundle By Name(w71) -> ("ACT Input"=w70:T28)
    n31 = call "Detect CMD Change.vi"("CMD_ACT_SwerveDrive_Data"=w72, "Preious ACT Input"=w70) -> ("New Command"=w69:bool)  [unwired: 9 in]
    n32 = global read "Global_SEN_Data Out.vi" "Sen_Pigeon_YawPitchRoll"() -> (w112:T48)
    n33 = global read "Global_SEN_Data Out.vi" "Sen_Pigeon_Tilt Data"() -> (w78:T37)
    n34 = global read "Global_SEN_Data Out.vi" "Sen_Pigeon_Running"() -> (w109:bool)
    n35 = Unbundle By Name(w72) -> ("Orientation Robot(t) Field(f)"=w114:bool)
    n36 = Not(x=w109) -> (.not. x?=w108:bool)
    n37 = Unbundle By Name(w112) -> ("Yaw"=w101:T20)
    "Yaw" <- w101
    n38 = Or(x=w114, y=w108) -> (x .or. y?=w110:bool)
    n39 = Select(t=T20 0.0, s=w110, f=w101) -> (s? t:f=w113:T20)
    n40 = Bundle By Name(cluster=w71, "New Cmd"=w69, "Stream"="Stream", "Previous Time"=w147, "Current Time"=w58, "ACT Input"=w72, "Drive Position Values"=w96, "Drive Velocity Values"=w63, "Drive Velocity Times"=w137, "Drive Output Times"=w135, "Drive Output Values"=w134, "Steer Position Values"=w130, "Compass Heading"=w113, "Tilt Data"=w78) -> (w62:T45)
    n41 = Unbundle By Name(w62) -> ("ACT Input"=w100:T28, "Rotation PID Config.PID Config"=w98:T3, "Compass Heading"=w97:T20)
    n42 = Unbundle By Name(w62) -> ("New Cmd"=w68:bool, "Drive Position Offsets"=w84:i32[], "Drive Position Values"=w85:i32[], "SwerveConfig.Drive.CPR"=w83:dbl, "SwerveConfig.Drive.Wheel Diameter (in)"=w82:dbl, "SwerveConfig.Drive.RevMotor/Wheel"=w81:dbl)
    n43 = Unbundle By Name(w62) -> ("Current Time"=w61:timestamp, "Previous Time"=w144:timestamp)
    "Current Time" <- w61
    n44 = flat-sequence {
      tunnel: w62 -> [_]
      tunnel: [w154] -> w60
      frame #0 {
        n45 = Get Date/Time In Seconds() -> (seconds since 1Jan1904=w154:timestamp)
      }
    }
    n46 = Unbundle By Name(w62) -> ("State"=w149:T1, "Previous State"=w146:T1)
    n47 = Subtract(x=w60, y=w61) -> (x-y=→"x-y":dbl)
    n48 = Subtract(x=w61, y=w144) -> (x-y=w64:dbl)
    n49 = global read "Global_STOP.vi" "STOP"() -> (w151:bool)
    n50 = call "Auto Angle.vi"("Yaw"=w97, "Rotation PID Config"=w98, "CMD_ACT_SwerveDrive_Data in"=w100) -> ("At Angle"=w88:bool, "CMD_ACT_SwerveDrive_Data out"=w99:T47)  [unwired: 7 in]
    n51 = call "Conver Encoder distance to ft.vi"("RevMotor/RevWheel"=w81, "New CMD"=w68, "Wheel Diameter (in)"=w82, "CPR (Ct/Rev Mot)"=w83, "Drive Position Values"=w85, "Drive Position Offsets"=w84) -> ("Calculated Ft Out"=w66:dbl, "Drive Position Offsets Out"=w67:i32[])  [unwired: 4 in]
    n52 = Bundle By Name(cluster=w62, "Drive Position Offsets"=w67, "Calculated Position (ft)"=w66, "ACT Input"=w99, "At Angle"=w88, "Cycle Time(S)"=w64) -> (w74:T45)
    n53 = Select(t=ENUM_ACT_State."Shutdown" ("State"), s=w151, f=w149) -> (s? t:f=w145:T1)
    "State" <- w145
    n54 = case shown="\"Configuring\"" w145 {
      selector: w145 -> [_ _ _ w529 _ _ w609 _ _]
      tunnel: w74 -> [w482 w488 w508 w532 w567 w577 w607 w634 w658]
      tunnel: [w483 w489 w509 w533 w566 w578 w612 w637 w658] -> w133
      tunnel: [ENUM_ACT_State."Configuring" ("State") w490 w510 w534 w564 w579 w613 w638 ENUM_ACT_State."Shutdown" ("State")] -> w152
      tunnel: [w485 w486 w506 w530 w565 w575 w610 w635 w656] -> w105
      tunnel: w146 -> [_ _ _ w528 _ _ w608 _ _]
      frame "Startup" {
        w485 = T46[] [enum."Reset Time", enum."Save Position Offsets"] items=["Set Move from Values", "Swerve Config Drive Read ", "Swerve Config Azimuth Read", "No Action", "Reset Time", "Set to Coast", "Record Data", "Swerve Open Only", "Swerve Config ALL Update", "Swerve Config Azimuth Update", "Swerve Config Drive Update", "Swerve Config From FP Update", "File Config ALL Save", "File Config ALL Read", "Save Position Offsets", "Drive Auto PID", "Balance", "Brake", "Lock"] ("Actions")
        n55 = call "File RIO_Get Team Folder.vi"() -> ("Team Files Folder"=w481:path)  [unwired: 10 in, 1 out]
        n56 = Bundle By Name(cluster=w482, "Team Folder"=w481) -> (w483:T45)
      }
      frame "Coasting" {
        n57 = Unbundle By Name(w488) -> ("ACT Input.Mode"=w487:T29)
        n58 = case shown="\"Lock Wheels\"" w487 {
          tunnel: [ENUM_ACT_State."Moving" ("State") ENUM_ACT_State."Moving" ("State") ENUM_ACT_State."Moving" ("State") ENUM_ACT_State."Balancing" ("State") ENUM_ACT_State."Coasting" ("State") ENUM_ACT_State."Braking" ("State") ENUM_ACT_State."Locking Wheels" ("State")] -> w490
          tunnel: [w491 w493 w495 w497 w500 w502 w504] -> w489
          tunnel: w488 -> [w491 w493 w495 w497 w500 w502 w504]
          tunnel: [_ _ _ _ w499 _ _] -> w486
          frame "Manual" {
          }
          frame "Auto Trans Auto Rotate" {
          }
          frame "Manual Trans Auto Rotate" {
          }
          frame "Balance" {
          }
          frame "Coast" {
            w499 = T46[] [enum."Set to Coast"] items=["Set Move from Values", "Swerve Config Drive Read ", "Swerve Config Azimuth Read", "No Action", "Reset Time", "Set to Coast", "Record Data", "Swerve Open Only", "Swerve Config ALL Update", "Swerve Config Azimuth Update", "Swerve Config Drive Update", "Swerve Config From FP Update", "File Config ALL Save", "File Config ALL Read", "Save Position Offsets", "Drive Auto PID", "Balance", "Brake", "Lock"] ("Actions")
          }
          frame "Stop Brake" {
          }
          frame "Lock Wheels" {
          }
        }
      }
      frame "Locking Wheels" {
        n59 = Unbundle By Name(w508) -> ("ACT Input.Mode"=w507:T29)
        n60 = case shown="\"Lock Wheels\"" w507 {
          tunnel: [ENUM_ACT_State."Moving" ("State") ENUM_ACT_State."Moving" ("State") ENUM_ACT_State."Moving" ("State") ENUM_ACT_State."Balancing" ("State") ENUM_ACT_State."Coasting" ("State") ENUM_ACT_State."Braking" ("State") ENUM_ACT_State."Locking Wheels" ("State")] -> w510
          tunnel: [w511 w513 w515 w517 w520 w522 w525] -> w509
          tunnel: w508 -> [w511 w513 w515 w517 w520 w522 w525]
          tunnel: [_ _ _ _ w519 _ w524] -> w506
          frame "Manual" {
          }
          frame "Auto Trans Auto Rotate" {
          }
          frame "Manual Trans Auto Rotate" {
          }
          frame "Balance" {
          }
          frame "Coast" {
            w519 = T46[] [enum."Set to Coast"] items=["Set Move from Values", "Swerve Config Drive Read ", "Swerve Config Azimuth Read", "No Action", "Reset Time", "Set to Coast", "Record Data", "Swerve Open Only", "Swerve Config ALL Update", "Swerve Config Azimuth Update", "Swerve Config Drive Update", "Swerve Config From FP Update", "File Config ALL Save", "File Config ALL Read", "Save Position Offsets", "Drive Auto PID", "Balance", "Brake", "Lock"] ("Actions")
          }
          frame "Stop Brake" {
          }
          frame "Lock Wheels" {
            w524 = T46[] [enum."Lock"] items=["Set Move from Values", "Swerve Config Drive Read ", "Swerve Config Azimuth Read", "No Action", "Reset Time", "Set to Coast", "Record Data", "Swerve Open Only", "Swerve Config ALL Update", "Swerve Config Azimuth Update", "Swerve Config Drive Update", "Swerve Config From FP Update", "File Config ALL Save", "File Config ALL Read", "Save Position Offsets", "Drive Auto PID", "Balance", "Brake", "Lock"] ("Actions")
          }
        }
      }
      frame "Autoing" {
        n61 = Not Equal?(x=w529, y=w528) -> (x != y?=w527:bool)
        n62 = Unbundle By Name(w532) -> ("ACT Input.Mode"=w531:T29)
        n63 = case shown="\"Lock Wheels\"" w531 {
          tunnel: [ENUM_ACT_State."Moving" ("State") ENUM_ACT_State."Autoing" ("State") ENUM_ACT_State."Braking" ("State") ENUM_ACT_State."Locking Wheels" ("State") ENUM_ACT_State."Moving" ("State") ENUM_ACT_State."Balancing" ("State") ENUM_ACT_State."Coasting" ("State")] -> w534
          tunnel: [w535 w538 w541 w543 w544 w546 w549] -> w533
          tunnel: w532 -> [w535 w538 w541 w543 w544 w546 w549]
          tunnel: [_ w537 _ _ _ _ w548] -> w530
          tunnel: w527 -> [_ _ _ _ _ _ _]
          frame "Manual" {
          }
          frame "Auto Trans Auto Rotate" {
            w537 = T46[] [enum."Drive Auto PID", enum."Set Move from Values"] items=["Set Move from Values", "Swerve Config Drive Read ", "Swerve Config Azimuth Read", "No Action", "Reset Time", "Set to Coast", "Record Data", "Swerve Open Only", "Swerve Config ALL Update", "Swerve Config Azimuth Update", "Swerve Config Drive Update", "Swerve Config From FP Update", "File Config ALL Save", "File Config ALL Read", "Save Position Offsets", "Drive Auto PID", "Balance", "Brake", "Lock"] ("Actions")
          }
          frame "Stop Brake" {
          }
          frame "Lock Wheels" {
          }
          frame "Manual Trans Auto Rotate" {
          }
          frame "Balance" {
          }
          frame "Coast" {
            w548 = T46[] [enum."Set to Coast"] items=["Set Move from Values", "Swerve Config Drive Read ", "Swerve Config Azimuth Read", "No Action", "Reset Time", "Set to Coast", "Record Data", "Swerve Open Only", "Swerve Config ALL Update", "Swerve Config Azimuth Update", "Swerve Config Drive Update", "Swerve Config From FP Update", "File Config ALL Save", "File Config ALL Read", "Save Position Offsets", "Drive Auto PID", "Balance", "Brake", "Lock"] ("Actions")
          }
        }
      }
      frame "Configuring" {
        n64 = Unbundle By Name(w567) -> ("Team Folder"=w557:path, "Azimuth Config"=w563:T12, "Drive Config"=w562:T17, "Specific Config"=w561:T9)
        n65 = call "Config_Build Name.vim"("Config First Name"=w563) -> ("Cfg file"=w558:string)  [unwired: 9 in, 1 out]
        n66 = call "Config_Build Name.vim"("Config First Name"=w562) -> ("Cfg file"=w559:string)  [unwired: 9 in, 1 out]
        n67 = call "Config_Build Name.vim"("Config First Name"=w561) -> ("Cfg file"=w560:string)  [unwired: 9 in, 1 out]
        n68 = Build Path(base path=w557, name or relative path=w560) -> (appended path=w555:path)
        n69 = call <vilib>:"Check if File or Folder Exists.vi"("path"=w555) -> ("file or folder exists?"=w553:bool)  [unwired: 8 in, 2 out]
        n70 = Build Path(base path=w557, name or relative path=w559) -> (appended path=w556:path)
        n71 = Build Path(base path=w557, name or relative path=w558) -> (appended path=w568:path)
        n72 = call <vilib>:"Check if File or Folder Exists.vi"("path"=w556) -> ("file or folder exists?"=w552:bool)  [unwired: 8 in, 2 out]
        n73 = call <vilib>:"Check if File or Folder Exists.vi"("path"=w568) -> ("file or folder exists?"=w554:bool)  [unwired: 8 in, 2 out]
        n74 = Compound Arithmetic op=AND(w554, w552, w553) -> (w551:bool)
        n75 = case shown="False" w551 {
          tunnel: w567 -> [w571 w574]
          tunnel: [w571 w574] -> w566
          tunnel: [w570 w573] -> w565
          tunnel: [ENUM_ACT_State."Configuring" ("State") ENUM_ACT_State."Moving" ("State")] -> w564
          frame False {
            w570 = T46[] [enum."Swerve Open Only", enum."Swerve Config Azimuth Read", enum."Swerve Config Drive Read ", enum."File Config ALL Save"] items=["Set Move from Values", "Swerve Config Drive Read ", "Swerve Config Azimuth Read", "No Action", "Reset Time", "Set to Coast", "Record Data", "Swerve Open Only", "Swerve Config ALL Update", "Swerve Config Azimuth Update", "Swerve Config Drive Update", "Swerve Config From FP Update", "File Config ALL Save", "File Config ALL Read", "Save Position Offsets", "Drive Auto PID", "Balance", "Brake", "Lock"] ("Actions")
            # "RIO Config File Not Found"
          }
          frame True {
            w573 = T46[] [enum."File Config ALL Read", enum."Swerve Config ALL Update", enum."Set to Coast"] items=["Set Move from Values", "Swerve Config Drive Read ", "Swerve Config Azimuth Read", "No Action", "Reset Time", "Set to Coast", "Record Data", "Swerve Open Only", "Swerve Config ALL Update", "Swerve Config Azimuth Update", "Swerve Config Drive Update", "Swerve Config From FP Update", "File Config ALL Save", "File Config ALL Read", "Save Position Offsets", "Drive Auto PID", "Balance", "Brake", "Lock"] ("Actions")
            # "RIO Config File Found"
          }
        }
      }
      frame "Moving" {
        n76 = Unbundle By Name(w577) -> ("ACT Input.Mode"=w576:T29)
        n77 = case shown="\"Lock Wheels\"" w576 {
          tunnel: [ENUM_ACT_State."Moving" ("State") ENUM_ACT_State."Braking" ("State") ENUM_ACT_State."Locking Wheels" ("State") ENUM_ACT_State."Autoing" ("State") ENUM_ACT_State."Moving" ("State") ENUM_ACT_State."Coasting" ("State") ENUM_ACT_State."Balancing" ("State")] -> w579
          tunnel: [w581 w583 w585 w587 w590 w594 w597] -> w578
          tunnel: w577 -> [w581 w583 w585 w587 w590 w594 w597]
          tunnel: [w580 _ _ w588 w591 w593 w596] -> w575
          frame "Manual" {
            w580 = T46[] [enum."Set Move from Values"] items=["Set Move from Values", "Swerve Config Drive Read ", "Swerve Config Azimuth Read", "No Action", "Reset Time", "Set to Coast", "Record Data", "Swerve Open Only", "Swerve Config ALL Update", "Swerve Config Azimuth Update", "Swerve Config Drive Update", "Swerve Config From FP Update", "File Config ALL Save", "File Config ALL Read", "Save Position Offsets", "Drive Auto PID", "Balance", "Brake", "Lock"] ("Actions")
          }
          frame "Stop Brake" {
          }
          frame "Lock Wheels" {
          }
          frame "Auto Trans Auto Rotate" {
            w588 = T46[] [enum."Set Move from Values"] items=["Set Move from Values", "Swerve Config Drive Read ", "Swerve Config Azimuth Read", "No Action", "Reset Time", "Set to Coast", "Record Data", "Swerve Open Only", "Swerve Config ALL Update", "Swerve Config Azimuth Update", "Swerve Config Drive Update", "Swerve Config From FP Update", "File Config ALL Save", "File Config ALL Read", "Save Position Offsets", "Drive Auto PID", "Balance", "Brake", "Lock"] ("Actions")
          }
          frame "Manual Trans Auto Rotate" {
            w591 = T46[] [enum."Set Move from Values"] items=["Set Move from Values", "Swerve Config Drive Read ", "Swerve Config Azimuth Read", "No Action", "Reset Time", "Set to Coast", "Record Data", "Swerve Open Only", "Swerve Config ALL Update", "Swerve Config Azimuth Update", "Swerve Config Drive Update", "Swerve Config From FP Update", "File Config ALL Save", "File Config ALL Read", "Save Position Offsets", "Drive Auto PID", "Balance", "Brake", "Lock"] ("Actions")
          }
          frame "Coast" {
            w593 = T46[] [enum."Set to Coast"] items=["Set Move from Values", "Swerve Config Drive Read ", "Swerve Config Azimuth Read", "No Action", "Reset Time", "Set to Coast", "Record Data", "Swerve Open Only", "Swerve Config ALL Update", "Swerve Config Azimuth Update", "Swerve Config Drive Update", "Swerve Config From FP Update", "File Config ALL Save", "File Config ALL Read", "Save Position Offsets", "Drive Auto PID", "Balance", "Brake", "Lock"] ("Actions")
          }
          frame "Balance" {
            w596 = T46[] [enum."Balance"] items=["Set Move from Values", "Swerve Config Drive Read ", "Swerve Config Azimuth Read", "No Action", "Reset Time", "Set to Coast", "Record Data", "Swerve Open Only", "Swerve Config ALL Update", "Swerve Config Azimuth Update", "Swerve Config Drive Update", "Swerve Config From FP Update", "File Config ALL Save", "File Config ALL Read", "Save Position Offsets", "Drive Auto PID", "Balance", "Brake", "Lock"] ("Actions")
          }
        }
      }
      frame "Balancing" {
        n78 = Not Equal?(x=w609, y=w608) -> (x != y?=w606:bool)
        n79 = Bundle By Name(cluster=w607, "Reset Balance"=w606) -> (w600:T45)
        n80 = Unbundle By Name(w600) -> ("Tilt Data.Tilt Changing"=w601:bool, "Tilt Data.BACK UP"=w604:bool, "Tilt Data.BACK DOWN"=w602:bool)
        n81 = Unbundle By Name(w600) -> ("ACT Input.Mode"=w611:T29)
        n82 = Or(x=w604, y=w602) -> (x .or. y?=w603:bool)
        n83 = Not(x=w603) -> (.not. x?=w605:bool)
        n84 = Or(x=w601, y=w605) -> (x .or. y?=w599:bool)
        n85 = case shown="\"Balance\"" w611 {
          tunnel: [ENUM_ACT_State."Moving" ("State") ENUM_ACT_State."Autoing" ("State") ENUM_ACT_State."Braking" ("State") ENUM_ACT_State."Locking Wheels" ("State") ENUM_ACT_State."Balancing" ("State") ENUM_ACT_State."Moving" ("State") ENUM_ACT_State."Coasting" ("State")] -> w613
          tunnel: [w615 w617 w619 w621 w626 w629 w632] -> w612
          tunnel: w600 -> [w615 w617 w619 w621 w626 w629 w632]
          tunnel: [w614 _ _ _ w624 _ w631] -> w610
          tunnel: w599 -> [_ _ _ _ w623 _ _]
          frame "Manual" {
            w614 = T46[] [enum."Set Move from Values"] items=["Set Move from Values", "Swerve Config Drive Read ", "Swerve Config Azimuth Read", "No Action", "Reset Time", "Set to Coast", "Record Data", "Swerve Open Only", "Swerve Config ALL Update", "Swerve Config Azimuth Update", "Swerve Config Drive Update", "Swerve Config From FP Update", "File Config ALL Save", "File Config ALL Read", "Save Position Offsets", "Drive Auto PID", "Balance", "Brake", "Lock"] ("Actions")
          }
          frame "Auto Trans Auto Rotate" {
          }
          frame "Stop Brake" {
          }
          frame "Lock Wheels" {
          }
          frame "Balance" {
            n86 = case shown="True" w623 {
              tunnel: [w627 w628] -> w624
              frame False {
                w627 = T46[] [enum."Balance", enum."Set Move from Values"] items=["Set Move from Values", "Swerve Config Drive Read ", "Swerve Config Azimuth Read", "No Action", "Reset Time", "Set to Coast", "Record Data", "Swerve Open Only", "Swerve Config ALL Update", "Swerve Config Azimuth Update", "Swerve Config Drive Update", "Swerve Config From FP Update", "File Config ALL Save", "File Config ALL Read", "Save Position Offsets", "Drive Auto PID", "Balance", "Brake", "Lock"] ("Actions")
                # "Tilted"
              }
              frame True {
                w628 = T46[] [enum."Lock", enum."Balance"] items=["Set Move from Values", "Swerve Config Drive Read ", "Swerve Config Azimuth Read", "No Action", "Reset Time", "Set to Coast", "Record Data", "Swerve Open Only", "Swerve Config ALL Update", "Swerve Config Azimuth Update", "Swerve Config Drive Update", "Swerve Config From FP Update", "File Config ALL Save", "File Config ALL Read", "Save Position Offsets", "Drive Auto PID", "Balance", "Brake", "Lock"] ("Actions")
                # "Level or Tilting"
              }
            }
          }
          frame "Manual Trans Auto Rotate" {
          }
          frame "Coast" {
            w631 = T46[] [enum."Set to Coast"] items=["Set Move from Values", "Swerve Config Drive Read ", "Swerve Config Azimuth Read", "No Action", "Reset Time", "Set to Coast", "Record Data", "Swerve Open Only", "Swerve Config ALL Update", "Swerve Config Azimuth Update", "Swerve Config Drive Update", "Swerve Config From FP Update", "File Config ALL Save", "File Config ALL Read", "Save Position Offsets", "Drive Auto PID", "Balance", "Brake", "Lock"] ("Actions")
          }
        }
      }
      frame "Braking" {
        n87 = Unbundle By Name(w634) -> ("ACT Input.Mode"=w636:T29)
        n88 = case shown="\"Lock Wheels\"" w636 {
          tunnel: [ENUM_ACT_State."Moving" ("State") ENUM_ACT_State."Autoing" ("State") ENUM_ACT_State."Braking" ("State") ENUM_ACT_State."Locking Wheels" ("State") ENUM_ACT_State."Balancing" ("State") ENUM_ACT_State."Moving" ("State") ENUM_ACT_State."Coasting" ("State")] -> w638
          tunnel: [w640 w642 w645 w647 w650 w651 w654] -> w637
          tunnel: w634 -> [w640 w642 w645 w647 w650 w651 w654]
          tunnel: [w639 _ w644 _ _ _ w653] -> w635
          frame "Manual" {
            w639 = T46[] [enum."Set Move from Values"] items=["Set Move from Values", "Swerve Config Drive Read ", "Swerve Config Azimuth Read", "No Action", "Reset Time", "Set to Coast", "Record Data", "Swerve Open Only", "Swerve Config ALL Update", "Swerve Config Azimuth Update", "Swerve Config Drive Update", "Swerve Config From FP Update", "File Config ALL Save", "File Config ALL Read", "Save Position Offsets", "Drive Auto PID", "Balance", "Brake", "Lock"] ("Actions")
          }
          frame "Auto Trans Auto Rotate" {
          }
          frame "Stop Brake" {
            w644 = T46[] [enum."Brake", enum."Set Move from Values"] items=["Set Move from Values", "Swerve Config Drive Read ", "Swerve Config Azimuth Read", "No Action", "Reset Time", "Set to Coast", "Record Data", "Swerve Open Only", "Swerve Config ALL Update", "Swerve Config Azimuth Update", "Swerve Config Drive Update", "Swerve Config From FP Update", "File Config ALL Save", "File Config ALL Read", "Save Position Offsets", "Drive Auto PID", "Balance", "Brake", "Lock"] ("Actions")
          }
          frame "Lock Wheels" {
          }
          frame "Balance" {
          }
          frame "Manual Trans Auto Rotate" {
          }
          frame "Coast" {
            w653 = T46[] [enum."Set to Coast"] items=["Set Move from Values", "Swerve Config Drive Read ", "Swerve Config Azimuth Read", "No Action", "Reset Time", "Set to Coast", "Record Data", "Swerve Open Only", "Swerve Config ALL Update", "Swerve Config Azimuth Update", "Swerve Config Drive Update", "Swerve Config From FP Update", "File Config ALL Save", "File Config ALL Read", "Save Position Offsets", "Drive Auto PID", "Balance", "Brake", "Lock"] ("Actions")
          }
        }
      }
      frame "Shutdown" {
        w656 = T46[] [enum."Set to Coast"] items=["Set Move from Values", "Swerve Config Drive Read ", "Swerve Config Azimuth Read", "No Action", "Reset Time", "Set to Coast", "Record Data", "Swerve Open Only", "Swerve Config ALL Update", "Swerve Config Azimuth Update", "Swerve Config Drive Update", "Swerve Config From FP Update", "File Config ALL Save", "File Config ALL Read", "Save Position Offsets", "Drive Auto PID", "Balance", "Brake", "Lock"] ("Actions")
      }
    }
    n89 = Build Array("Read Saved Config", "Update Config", "Reset Distance") -> (w92:bool[])
    n90 = Or Array Elements(Boolean array=w92) -> (logical OR=w93:bool)
    n91 = case shown="True" w93 {
      tunnel: [_ w184] -> w75
      tunnel: w92 -> [_ w183]
      frame False {
      }
      frame True {
        n92 = call "Search Unsorted 1D Array.vim"("element"=TRUE, "unsorted 1D array"=w183) -> ("index of element"=w181:i32)  [unwired: 9 in]
        n93 = case shown="1" w181 {
          tunnel: [w185 w186 w187] -> w184
          frame ..0 {
            w185 = T46[] [enum."File Config ALL Read"] items=["Set Move from Values", "Swerve Config Drive Read ", "Swerve Config Azimuth Read", "No Action", "Reset Time", "Set to Coast", "Record Data", "Swerve Open Only", "Swerve Config ALL Update", "Swerve Config Azimuth Update", "Swerve Config Drive Update", "Swerve Config From FP Update", "File Config ALL Save", "File Config ALL Read", "Save Position Offsets", "Drive Auto PID", "Balance", "Brake", "Lock"] ("Actions")
          }
          frame 1 {
            w186 = T46[] [enum."Swerve Config From FP Update", enum."Swerve Config ALL Update", enum."File Config ALL Save"] items=["Set Move from Values", "Swerve Config Drive Read ", "Swerve Config Azimuth Read", "No Action", "Reset Time", "Set to Coast", "Record Data", "Swerve Open Only", "Swerve Config ALL Update", "Swerve Config Azimuth Update", "Swerve Config Drive Update", "Swerve Config From FP Update", "File Config ALL Save", "File Config ALL Read", "Save Position Offsets", "Drive Auto PID", "Balance", "Brake", "Lock"] ("Actions")
          }
          frame 2.. {
            w187 = T46[] [enum."Save Position Offsets"] items=["Set Move from Values", "Swerve Config Drive Read ", "Swerve Config Azimuth Read", "No Action", "Reset Time", "Set to Coast", "Record Data", "Swerve Open Only", "Swerve Config ALL Update", "Swerve Config Azimuth Update", "Swerve Config Drive Update", "Swerve Config From FP Update", "File Config ALL Save", "File Config ALL Read", "Save Position Offsets", "Drive Auto PID", "Balance", "Brake", "Lock"] ("Actions")
          }
        }
      }
    }
    n94 = Unbundle By Name(w133) -> ("Stream"=w132:bool)
    n95 = Build Array (concatenate)(w75, w105) -> (w104:T46[])
    n96 = case shown="False" w132 {
      tunnel: w104 -> [w240 w243]
      tunnel: [w240 w242] -> w131
      frame False {
      }
      frame True {
        n97 = Build Array (concatenate)(w243, ENUM_ACT_Action."Record Data" ("Action")) -> (w242:T46[])
      }
    }
    n98 = Bundle By Name(cluster=w133, "Previous State"=w145, "State"=w152) -> (w153:T45)
    n99 = for {
      tunnel: w131 -> [w246] mode=indexing
      shift-right: [w245] -> w79
      shift-left: w153 -> [w244]
      n100 = case shown="\"Save Position Offsets\"" w246 {
        tunnel: w244 -> [w248 w277 w288 w294 w299 w302 w308 w332 w338 w357 w383 w395 w419 w435 w452 w456 w467 w472 w474]
        tunnel: [w267 w282 w289 w295 w299 w301 w310 w332 w337 w358 w382 w394 w420 w434 w451 w457 w466 w471 w480] -> w245
        frame "Set Move from Values" {
          w251 = 16.0  # Max Module Speed (ft/s)
          w254 = T19 2 items=["PercentOutput"=0, "Position"=1, "Velocity"=2, "Current"=3, "Follower"=5, "MotionProfile"=6, "MotionMagic"=7, "MotionProfileArc"=10, "Disabled"=15] ("Drive Control Mode")
          n101 = flat-sequence {
            tunnel: w248 -> [w271]
            tunnel: [w270] -> w256
            tunnel: [w269] -> w258
            tunnel: [w268] -> w253
            frame #0 {
              n102 = Unbundle By Name(w271) -> ("ACT Input.Direction"=w270:T30, "ACT Input.Rotation Reduction 1-0"=w268:dbl)
              n103 = call <vilib>:"High Resolution Relative Seconds.vi"() -> ("relative seconds"=w269:dbl)
            }
          }
          n104 = Unbundle By Name(w248) -> ("Swerve Set"=w261:T24, "SwerveConfig.Frame"=w259:T33, "Compass Heading"=w255:T20, "ACT Input.Rotation Center From Robot Center"=w252:T32)
          n105 = Unbundle By Name(w248) -> ("SwerveConfig.Drive.RevMotor/Wheel"=w263:dbl, "SwerveConfig.Drive.Wheel Diameter (in)"=w264:dbl, "ACT Input.Max Translation Speed (ft/sec)"=w249:dbl)
          "Max Tranlation FPS" <- w249
          n106 = Unbundle By Name(w248) -> ("SwerveConfig.Drive.CPR"=w247:dbl)
          n107 = Divide(x=w249, y=w251) -> (x/y=w250:dbl)
          n108 = call "Convert to Field  Orientation.vi"("Compass Heading"=w255, "Direction in"=w256) -> ("Corrected Direction out"=w257:T30)  [unwired: 9 in]
          n109 = call "Swerve Calculate Angle and Velocity.vi"("Max Translation Output(0-1)"=w250, "Rotation Reduction"=w253, "Frame"=w259, "Rotation Center From Robot Center"=w252, "Comand Data"=w257) -> ("Swerve Request Out"=w262:T24)  [unwired: 6 in]
          n110 = call "Convert FPS to CP100ms.vi"("RevMotor/RevWheel"=w263, "Wheel Diameter (in)"=w264, "CPR"=w247, "Translation Speed (ft/s)"=w251) -> ("Motor Speed (Counts/100ms) Out"=w265:dbl)  [unwired: 7 in]
          n111 = call "Optomize Settings.vi"("Previous Swerve Setting"=w261, "Swerve Request"=w262) -> ("Swerve Setting Out"=w260:T24)  [unwired: 9 in]
          n112 = Bundle By Name(cluster=w248, "Steer Mode"=ENUM_Steer_Mode_Select."Steer", "Swerve Set"=w260, "Max Velocity CP100ms"=w265, "Drive Control Mode"=w254, "calc Start Time"=w258) -> (w267:T45)
        }
        frame "Lock" {
          w272 = T26 0.0 ("Front Right.Velocity")
          w273 = T20 0.125 ("Front Left.Angle")
          w274 = T20 0.875 ("Front Right.Angle")
          w279 = T19 2 items=["PercentOutput"=0, "Position"=1, "Velocity"=2, "Current"=3, "Follower"=5, "MotionProfile"=6, "MotionMagic"=7, "MotionProfileArc"=10, "Disabled"=15] ("Drive Control Mode")
          n113 = Unbundle By Name(w277) -> ("Swerve Set"=w276:T24)
          n114 = Bundle By Name(cluster=w276, "Front Right.Angle"=w274, "Front Left.Angle"=w273, "Back Left.Angle"=w274, "Back Right.Angle"=w273, "Front Right.Velocity"=w272, "Front Left.Velocity"=w272, "Back Left.Velocity"=w272, "Back Right.Velocity"=w272) -> (w275:T24)
          n115 = call <vilib>:"High Resolution Relative Seconds.vi"() -> ("relative seconds"=w280:dbl)
          n116 = Bundle By Name(cluster=w277, "Steer Mode"=ENUM_Steer_Mode_Select."Steer", "Swerve Set"=w275, "Max Velocity CP100ms"=0.0, "Drive Control Mode"=w279, "calc Start Time"=w280) -> (w282:T45)
        }
        frame "Swerve Config Drive Read " {
          n117 = Unbundle By Name(w288) -> ("Drive Refs"=w290:T40[], "Drive Config"=w286:T17)
          n118 = Index Array(array=w290) -> (element=w287:T40)  [unwired: 1 in]
          n119 = call "Swerve_Module Drive Read Config.vi"("Send Cmd Timout(ms)"=u32 300, "Module Drive Config Data"=w286, "PhoenixMotorControlDevRef"=w287) -> ("Module Azimuth Config Data Out"=w284:T17)  [unwired: 6 in, 2 out]
          n120 = Bundle By Name(cluster=w288, "Drive Config"=w284, "Update Display"=TRUE) -> (w289:T45)
        }
        frame "Swerve Config Azimuth Read" {
          n121 = Unbundle By Name(w294) -> ("Steer Refs"=w298:T40[], "Azimuth Config"=w296:T12)
          n122 = Index Array(array=w298) -> (element=w297:T40)  [unwired: 1 in]
          n123 = call "Swerve_Module Azimuth Read Config.vi"("Send Cmd Timout(ms)"=u32 300, "Module Azimuth Config Data"=w296, "PhoenixMotorControlDevRef"=w297) -> ("Module Azimuth Config Data Out"=w292:T12)  [unwired: 6 in, 2 out]
          n124 = Bundle By Name(cluster=w294, "Azimuth Config"=w292, "Update Display"=TRUE) -> (w295:T45)
        }
        frame "No Action" {
        }
        frame "Reset Time" {
          # "Reset timer by taking the current time\nand making it the start time\n\nLater when the current time is \nsubtracted from the start time\nyou will get the elapsed time in \nseconds"
          n125 = Unbundle By Name(w302) -> ("Current Time"=w300:timestamp)
          n126 = Bundle By Name(cluster=w302, "Start Time"=w300) -> (w301:T45)
        }
        frame "Set to Coast" {
          w303 = T19 0 items=["PercentOutput"=0, "Position"=1, "Velocity"=2, "Current"=3, "Follower"=5, "MotionProfile"=6, "MotionMagic"=7, "MotionProfileArc"=10, "Disabled"=15] ("Drive Control Mode")
          n127 = Unbundle By Name(w308) -> ("Motor List"=w306:T11[], "Swerve Set"=w305:T24)
          n128 = for {
            tunnel: w306 -> [w313] mode=indexing
            shift-right: [w311] -> w304
            shift-left: w305 -> [w312]
            n129 = case shown="\"Left-Back\"" w313 {
              tunnel: w312 -> [w316 w319 w322 w325]
              tunnel: [w315 w318 w321 w324] -> w311
              frame "Right-Front" {
                n130 = Bundle By Name(cluster=w316, "Front Right.Velocity"=T26 0.0 ("Front Right.Velocity (0-1)")) -> (w315:T24)
              }
              frame "Left-Back" {
                n131 = Bundle By Name(cluster=w319, "Back Left.Velocity"=T26 0.0 ("Front Right.Velocity (0-1)")) -> (w318:T24)
              }
              frame "Right-Back" {
                n132 = Bundle By Name(cluster=w322, "Back Right.Velocity"=T26 0.0 ("Front Right.Velocity (0-1)")) -> (w321:T24)
              }
              frame "Left-Front" {
                n133 = Bundle By Name(cluster=w325, "Front Left.Velocity"=T26 0.0 ("Front Right.Velocity (0-1)")) -> (w324:T24)
              }
            }
          }
          n134 = Bundle By Name(cluster=w308, "Swerve Set"=w304, "Drive Control Mode"=w303, "Drive PID Slot"=0, "Steer Mode"=ENUM_Steer_Mode_Select."Off") -> (w310:T45)
        }
        frame "Record Data" {
          n135 = Unbundle By Name(w332) -> ("Motor List"=w326:T11[], "Drive Velocity Times"=w331:dbl[], "Drive Velocity Values"=w330:dbl[], "Steer Position Values"=w329:dbl[], "Drive Output Times"=w328:dbl[], "Drive Output Values"=w327:dbl[])
          n136 = call "Stream ALL Velocity Values.vi"("Output Values"=w327, "Motor List"=w326, "Output Times"=w328, "Drive Target Values"=w329, "Drive Velocity Values"=w330, "Drive Times"=w331) -> ()  [unwired: 6 in]
        }
        frame "Swerve Open Only" {
          n137 = Unbundle By Name(w338) -> ("Specific Config.Data"=w336:T10[])
          n138 = for {
            tunnel: w336 -> [w348] mode=indexing
            tunnel: [w346] -> w335 mode=indexing
            tunnel: [w345] -> w334 mode=indexing
            tunnel: [w344] -> w333 mode=indexing
            tunnel: [w341] -> _ mode=indexing
            tunnel: [w340] -> _ mode=indexing
            tunnel: [w339] -> _ mode=indexing
            n139 = Unbundle By Name(w348) -> ("CAN Bus"=w347:string, "Drive ID"=w349:u8, "Azimuth ID"=w343:u8, "CanCoder ID"=w342:u8)
            n140 = call <vilib>:"CTRE_Phoenix_TalonFX_Open.vi"("Device Number"=w349, "CAN Bus"=w347) -> ("error out"=w339:errorcluster, "PhoenixMotorControlDevRef"=w346:T40)  [unwired: 8 in]
            n141 = call <vilib>:"CTRE_Phoenix_TalonFX_Open.vi"("Device Number"=w343, "CAN Bus"=w347) -> ("error out"=w340:errorcluster, "PhoenixMotorControlDevRef"=w345:T40)  [unwired: 8 in]
            n142 = call <vilib>:"CTRE_Phoenix_CANcoder_Open.vi"("Device Number"=w342, "CAN Bus"=w347) -> ("error out"=w341:errorcluster, "CTRE_CANcoder_DeviceRef"=w344:T39)  [unwired: 8 in]
          }
          n143 = Bundle By Name(cluster=w338, "Drive Refs"=w335, "Steer Refs"=w334, "CANCoder Refs"=w333) -> (w337:T45)
        }
        frame "Swerve Config ALL Update" {
          n144 = Unbundle By Name(w357) -> ("Specific Config.Data"=w356:T10[], "Drive Config"=w353:T17, "Azimuth Config"=w354:T12)
          n145 = for {
            tunnel: [w365] -> w351 mode=indexing
            tunnel: [w363] -> w352 mode=indexing
            tunnel: [w366] -> w350 mode=indexing
            tunnel: w356 -> [w362] mode=indexing
            tunnel: [w364] -> w355 mode=indexing
            tunnel: w353 -> [w360]
            tunnel: w354 -> [w359]
            n146 = case shown="True" FALSE {
              tunnel: [w372 w379] -> w366
              tunnel: [w371 w378] -> w365
              tunnel: [w373 w377] -> w364
              tunnel: [w370 w376] -> w363
              tunnel: w362 -> [w374 w375]
              tunnel: w360 -> [w369 _]
              tunnel: w359 -> [w368 _]
              frame False {
                n147 = call "Swerve_Module Config.vi"("Reset Config"=TRUE, "Module Unique Config Data"=w374, "Azimuth Config Data"=w368, "Drive Config Data"=w369) -> ("Drive Motor Ref Out"=w370:T40, "Azimuth Motor Ref Out"=w371:T40, "CANcoder Ref Out"=w372:T39)  [unwired: 4 in, 1 out]
                n148 = Unbundle By Name(w374) -> ("Motor Pos"=w373:T11)
              }
              frame True {
                n149 = call "Swerve_Simple Config.vi"("Module Azimuth Config Data"=w375) -> (0:"PhoenixMotorControlDevRef Out"=w376:T40, 1:"PhoenixMotorControlDevRef Out"=w378:T40, "CTRE_CANcoder_DeviceRef Out"=w379:T39, "Motor Pos Out"=w377:T11)  [unwired: 7 in]
              }
            }
          }
          n150 = Bundle By Name(cluster=w357, "Motor List"=w355, "CANCoder Refs"=w350, "Steer Refs"=w351, "Drive Refs"=w352) -> (w358:T45)
        }
        frame "Swerve Config Azimuth Update" {
          n151 = Unbundle By Name(w383) -> ("Specific Config.Data"=w380:T10[], "Steer Refs"=w385:T40[], "Azimuth Config"=w381:T12)
          n152 = for {
            tunnel: w385 -> [w390] mode=indexing
            tunnel: w381 -> [w389]
            tunnel: [w388] -> w384 mode=indexing
            tunnel: w380 -> [w386] mode=indexing
            n153 = call "Swerve_Module Azimuth Config.vi"("Max # Of Tries"=3, "Send Cmd Timout(ms)"=u32 300, "Specific Data"=w386, "Module Azimuth Config Data"=w389, "PhoenixMotorControlDevRef"=w390) -> ("Module Azimuth Ref Out"=w388:T40)  [unwired: 5 in, 1 out]
          }
          n154 = Bundle By Name(cluster=w383, "Steer Refs"=w384) -> (w382:T45)
        }
        frame "Swerve Config Drive Update" {
          n155 = Unbundle By Name(w395) -> ("Specific Config.Data"=w392:T10[], "Drive Refs"=w397:T40[], "Drive Config"=w393:T17)
          n156 = for {
            tunnel: w397 -> [w402] mode=indexing
            tunnel: w393 -> [w401]
            tunnel: [w400] -> w396 mode=indexing
            tunnel: w392 -> [w398] mode=indexing
            n157 = call "Swerve_Module Drive Config.vi"("Max # Of Tries"=3, "Send Cmd Timout(ms)"=u32 300, "Module Specific Data"=w398, "Module Drive Config Data"=w401, "PhoenixMotorControlDevRef"=w402) -> ("PhoenixMotorControlDevRef Out Out"=w400:T40)  [unwired: 5 in, 1 out]
          }
          n158 = Bundle By Name(cluster=w395, "Drive Refs"=w396) -> (w394:T45)
        }
        frame "Swerve Config From FP Update" {
          n159 = Unbundle By Name(w419) -> ("Current Time"=w418:timestamp)
          n160 = call "Date Stamp.vi"("Time"=w418) -> ("U64 Out"=w404:u64)  [unwired: 5 in, 1 out]
          n161 = Bundle By Name(cluster="Azimuth Config Data", "ModuleAzimuth Ver"=w404) -> (w412:T12)
          n162 = Bundle By Name(cluster="Auto PID Config", "AutoDrivePID Ver"=w404) -> (w407:T8)
          n163 = Bundle By Name(cluster="Auto Rotate Config", "AutoRotatePID Ver"=w404) -> (w409:T7)
          n164 = Bundle By Name(cluster="Balance Config", "BalancePID Ver"=w404) -> (w405:T2)
          n165 = Bundle By Name(cluster="Drive Config Data", "ModuleDrive Ver"=w404) -> (w414:T17)
          n166 = Bundle By Name(cluster="Module Specific Data", "SpecificData Ver"=w404) -> (w416:T9)
          n167 = Bundle By Name(cluster=w419, "Specific Config"=w416, "Drive Config"=w414, "Azimuth Config"=w412, "Update Display"=TRUE, "Rotation PID Config"=w409, "Auto PID Config"=w407, "Balance Config"=w405) -> (w420:T45)
        }
        frame "File Config ALL Save" {
          w421 = TRUE ("Read(f) Write(t)")
          n168 = Unbundle By Name(w435) -> ("Team Folder"=w422:path, "Specific Config"=w437:T9, "Azimuth Config"=w433:T12, "Drive Config"=w430:T17, "Rotation PID Config"=w426:T7, "Auto PID Config"=w425:T8, "Balance Config"=w424:T2)
          n169 = call "RWA_File Config.vim"("Read(f) Write(t)"=w421, "Target Folder Folder"=w422, "Any Config"=w437) -> ("Any Config Out"=w436:T9)  [unwired: 4 in, 4 out]
          n170 = call "RWA_File Config.vim"("Read(f) Write(t)"=w421, "Target Folder Folder"=w422, "Any Config"=w433) -> ("Any Config Out"=w431:T12)  [unwired: 4 in, 4 out]
          n171 = call "RWA_File Config.vim"("Read(f) Write(t)"=w421, "Target Folder Folder"=w422, "Any Config"=w430) -> ("Any Config Out"=w429:T17)  [unwired: 4 in, 4 out]
          n172 = call "RWA_File Config.vim"("Read(f) Write(t)"=w421, "Target Folder Folder"=w422, "Any Config"=w426) -> ("Any Config Out"=w428:T7)  [unwired: 4 in, 4 out]
          n173 = call "RWA_File Config.vim"("Read(f) Write(t)"=w421, "Target Folder Folder"=w422, "Any Config"=w425) -> ("Any Config Out"=w427:T8)  [unwired: 4 in, 4 out]
          n174 = call "RWA_File Config.vim"("Read(f) Write(t)"=w421, "Target Folder Folder"=w422, "Any Config"=w424) -> ("Any Config Out"=w423:T2)  [unwired: 4 in, 4 out]
          n175 = Bundle By Name(cluster=w435, "Specific Config"=w436, "Azimuth Config"=w431, "Drive Config"=w429, "Update Display"=TRUE, "Rotation PID Config"=w428, "Auto PID Config"=w427, "Balance Config"=w423) -> (w434:T45)
        }
        frame "File Config ALL Read" {
          w438 = FALSE ("Read(f) Write(t)")
          n176 = Unbundle By Name(w452) -> ("Team Folder"=w439:path, "Specific Config"=w454:T9, "Azimuth Config"=w450:T12, "Drive Config"=w449:T17, "Rotation PID Config"=w445:T7, "Auto PID Config"=w442:T8, "Balance Config"=w441:T2)
          n177 = call "RWA_File Config.vim"("Read(f) Write(t)"=w438, "Target Folder Folder"=w439, "Any Config"=w454) -> ("Any Config Out"=w453:T9)  [unwired: 4 in, 4 out]
          n178 = call "RWA_File Config.vim"("Read(f) Write(t)"=w438, "Target Folder Folder"=w439, "Any Config"=w450) -> ("Any Config Out"=w446:T12)  [unwired: 4 in, 4 out]
          n179 = call "RWA_File Config.vim"("Read(f) Write(t)"=w438, "Target Folder Folder"=w439, "Any Config"=w449) -> ("Any Config Out"=w447:T17)  [unwired: 4 in, 4 out]
          n180 = call "RWA_File Config.vim"("Read(f) Write(t)"=w438, "Target Folder Folder"=w439, "Any Config"=w445) -> ("Any Config Out"=w444:T7)  [unwired: 4 in, 4 out]
          n181 = call "RWA_File Config.vim"("Read(f) Write(t)"=w438, "Target Folder Folder"=w439, "Any Config"=w442) -> ("Any Config Out"=w443:T8)  [unwired: 4 in, 4 out]
          n182 = call "RWA_File Config.vim"("Read(f) Write(t)"=w438, "Target Folder Folder"=w439, "Any Config"=w441) -> ("Any Config Out"=w440:T2)  [unwired: 4 in, 4 out]
          n183 = Bundle By Name(cluster=w452, "Specific Config"=w453, "Azimuth Config"=w446, "Drive Config"=w447, "Update Display"=TRUE, "Rotation PID Config"=w444, "Auto PID Config"=w443, "Balance Config"=w440) -> (w451:T45)
        }
        frame "Save Position Offsets" {
          n184 = Unbundle By Name(w456) -> ("Drive Position Values"=w455:i32[])
          n185 = Bundle By Name(cluster=w456, "Drive Position Offsets"=w455) -> (w457:T45)
        }
        frame "Drive Auto PID" {
          n186 = Unbundle By Name(w467) -> ("Auto PID Config.PID Config"=w459:T3)
          n187 = Unbundle By Name(w467) -> ("Calculated Position (ft)"=w468:dbl, "ACT Input.Auto Target (ft)"=w464:dbl)
          n188 = call "Auto PID Drive.vi"("PID Config"=w459, "Auto Target (ft)"=w464, "Calculated Position (ft)"=w468, "Target Cycle Time(S)"=0.05) -> ("PID Enabled Out"=→"PID Enabled":bool, "Error Out"=→"Auto Drive error":dbl, "At Target"=w463:bool, "Output Out"=w461:dbl)  [unwired: 4 in]
          "At Target" <- w463
          "Velocity Out" <- w461
          n189 = Bundle By Name(cluster=w467, "ACT Input.Direction.Traverse.Angle"=T20 0.0, "ACT Input.Direction.Traverse.Velocity"=w461, "At Position"=w463) -> (w466:T45)
        }
        frame "Brake" {
          n190 = Bundle By Name(cluster=w472, "ACT Input.Direction.Traverse.Angle"=T20 0.0, "ACT Input.Direction.Traverse.Velocity"=T26 0.0) -> (w471:T45)
        }
        frame "Balance" {
          n191 = Unbundle By Name(w474) -> ("ACT Input.Auto Target (ft)"=w473:dbl)
          n192 = Unbundle By Name(w474) -> ("Tilt Data"=w476:T37, "Balance Config.PID"=w478:T3)
          n193 = call "Swerve Balance To Level PID.vi"("Yaw Data"=w476, "Position ft"=w473, "Tilt PID Config"=w478) -> ("Balanced"=w475:bool, "Output Cluster Out"=w479:T25)  [unwired: 6 in, 1 out]
          n194 = Bundle By Name(cluster=w474, "ACT Input.Direction.Traverse"=w479, "Reset Balance"=FALSE, "Balanced"=w475) -> (w480:T45)
        }
      }
    }
    n195 = Unbundle By Name(w79) -> ("Steer Refs"=w140:T40[], "Swerve Set"=w115:T24, "Motor List"=w123:T11[], "Steer Mode"=w127:T27, "SwerveConfig.Steer.CPR"=w124:dbl, "Max Velocity CP100ms"=w125:dbl, "Drive Refs"=w139:T40[], "Drive Control Mode"=w126:T19, "Drive PID Slot"=w107:i32)
    "Steer Mode" <- w127
    "Max Velocity(CP100ms)" <- w125
    "Swerve Set" <- w115
    "Drive Control Mode" <- w126
    n196 = Unbundle By Name(w79) -> ("Cycle Time(S)"=w141:dbl)
    "Cycle Time (S)" <- w141
    n197 = Unbundle By Name(w79) -> ("Drive Position Values"=w91:i32[], "Drive Position Offsets"=w90:i32[])
    n198 = Unbundle By Name(w79) -> ("Calculated Position (ft)"=w65:dbl)
    "Calculated Position ft" <- w65
    n199 = Unbundle By Name(w79) -> ("ACT Input"=→"Input CMD":T28)
    n200 = disable-structure shown="Disabled" {
      disable-tunnel: w79 -> [w167 _]
      frame Disabled {
        n201 = Unbundle By Name(w167) -> ("Steer Position Values"=w166:dbl[], "SwerveConfig.Drive.RevMotor/Wheel"=w168:dbl, "SwerveConfig.Drive.Wheel Diameter (in)"=w169:dbl, "Drive Position Values"=w171:i32[], "Drive Position Offsets"=w170:i32[], "SwerveConfig.Drive.CPR"=w172:dbl)
        n202 = Index Array(array=w166, index #1=1 ("index"), index #2=0 ("index"), index #3=2 ("index"), index #4=3 ("index")) -> (element #1=w161:dbl, element #2=w160:dbl, element #3=w159:dbl, element #4=w158:dbl)
        n203 = Build Array(w161, w160, w159, w158) -> (w156:dbl[])
        n204 = for {
          tunnel: [w177] -> w173 mode=indexing
          tunnel: w171 -> [w180] mode=indexing
          tunnel: w170 -> [w179] mode=indexing
          tunnel: w172 -> [w176]
          tunnel: w169 -> [w175]
          tunnel: w168 -> [w174]
          n205 = Subtract(x=w180, y=w179) -> (x-y=w178:i32)
          n206 = call "Convert Counts to Feet.vi"("RevMotor/RevWheel"=w174, "Wheel Diameter (in)"=w175, "CPR (Ct/Rev mot)"=w176, "Counts"=w178) -> ("Ft"=w177:dbl)  [unwired: 7 in]
        }
        n207 = Multiply(x=w156, y=360.0 ("Numeric")) -> (x*y=w155:dbl[])
        n208 = global write "Global_ACT_Data Out.vi" "ACT_SwerveDrive_Directions"(w155) -> ()
        n209 = global write "Global_ACT_Data Out.vi" "ACT_Drive_Distances_(ft)"(w173) -> ()
      }
      frame Enabled {
      }
    }
    n210 = Unbundle By Name(w79) -> ("At Position"=w87:bool, "At Angle"=w86:bool, "Balanced"=w77:bool)
    "At Position" <- w87
    "At Angle" <- w86
    "Balanced" <- w77
    n211 = Subtract(x=w91, y=w90) -> (x-y=→"Calculated Position Values":i32[])
    n212 = global write "Global_ACT_Data Out.vi" "ACT_Swerve_Position ft"(w65) -> ()
    n213 = global write "Global_ACT_Data Out.vi" "ACT_SwerveDrive_Balanced"(w77) -> ()
    n214 = Unbundle By Name(w79) -> ("Update Display"=w102:bool)
    n215 = global write "Global_ACT_Data Out.vi" "ACT_Swerve_CycleTime(S)"(w141) -> ()
    n216 = global write "Global_ACT_Data Out.vi" "ACT_SwerveDrive_At Position"(w87) -> ()
    n217 = global write "Global_ACT_Data Out.vi" "ACT_SwerveDrive_At Angle"(w86) -> ()
    n218 = call "Set Steer Motors.vi"("Disable"=w76, "PPR"=w124, "Offset Encoder Positions"=dbl[] [0.0, 0.0, 0.0, 0.0], "Steer Control Mode"=w127, "Motor List"=w123, "Swerve Data"=w115, "Steer Refs"=w140) -> ("Encoder Counts Out"=w117:dbl[], "Array Out"=w122:T40[])  [unwired: 3 in]
    n219 = call "Set Drive Motors.vi"("Disable"=w119, "Drive PID Slot"=w107, "Max Velocity(CP100ms)"=w125, "Control Mode"=w126, "Motor List"=w123, "Swerve Data"=w115, "Drive Refs"=w139) -> ("Speeds"=w116:dbl[], "Array Out"=w138:T40[])  [unwired: 3 in]
    n220 = case shown="True" w102 {
      tunnel: w79 -> [_ w189]
      frame False {
      }
      frame True {
        n221 = Unbundle By Name(w189) -> ("Rotation PID Config"=w190:T7)
        n222 = Unbundle By Name(w189) -> ("Auto PID Config"=w188:T8)
        n223 = Unbundle By Name(w189) -> ("Specific Config"=w193:T9)
        n224 = Unbundle By Name(w189) -> ("Drive Config"=w191:T17)
        n225 = Unbundle By Name(w189) -> ("Azimuth Config"=w192:T12)
        n226 = local write "Module Specific Data"(w193) -> ()
        n227 = local write "Azimuth Config Data"(w192) -> ()
        n228 = local write "Auto Rotate Config"(w190) -> ()
        n229 = local write "Auto PID Config"(w188) -> ()
        n230 = local write "Drive Config Data"(w191) -> ()
      }
    }
    n231 = flat-sequence {
      tunnel: w122 -> [w198]
      tunnel: [w198] -> w121
      tunnel: w79 -> [w197]
      tunnel: [w197] -> w120
      frame #0 {
        n232 = Unbundle By Name(w197) -> ("calc Start Time"=w195:dbl)
        n233 = call <vilib>:"High Resolution Relative Seconds.vi"() -> ("relative seconds"=w196:dbl)
        n234 = Subtract(x=w196, y=w195) -> (x-y=→"calc time":dbl)
      }
    }
    n235 = feedback #1() -> (w118:T21)  [unwired: 1 in]
    n236 = call "Build Actual View.vi"("Encoder Counts Out"=w117, "Speeds"=w116, "Previous Actual"=w118, "Swerve Set"=w115) -> ("Swerve Data out"=w80:T21)  [unwired: 7 in]
    "Swerve SET Actual" <- w80
    n237 = feedback-in #1(w80) -> ()
    n238 = Bundle By Name(cluster=w120, "Update Display"=FALSE, "Steer Refs"=w121, "Drive Refs"=w138) -> (w142:T45)
  }
  n239 = flat-sequence {
    frame #0 {
      (unwired) ENUM_Swerve_CMD_Mode_Select."Coast" ("ACT Input.Mode")
      (unwired) ENUM_ACT_State."Startup" ("State")
      (unwired) ENUM_ACT_Action."Swerve Config Drive Read " ("Action")
      # "mode"
      # "State LIST"
      # "Action LIST"
    }
  }
  n240 = Unbundle By Name(w49) -> ("Drive Refs"=w44:T40[], "Steer Refs"=w45:T40[])  [unwired: 1 out]
  n241 = for {
    tunnel: w45 -> [w659] mode=indexing
    tunnel: w44 -> [w660] mode=indexing
    n242 = call <vilib>:"WPI_MotorControlClose.vi"("MotorControlDevRef"=w659) -> ()  [unwired: 10 in, 1 out]
    n243 = call <vilib>:"WPI_MotorControlClose.vi"("MotorControlDevRef"=w660) -> ()  [unwired: 10 in, 1 out]
  }
